vi "界面3.vi"() -> ()   [LabVIEW 2014]
uses:
  <vilib>/Analysis/3filter.llb/Filter Passband Type.ctl
  <vilib>/Analysis/4window.llb/windowTd.ctl
  <vilib>/Platform/TimedLoop/XDataNode/timing_clust.ctl
  <vilib>/Platform/TimedLoop/XDataNode/nitl_modes.ctl
  <vilib>/Platform/TimedLoop/XDataNode/wakeup.ctl
  <vilib>/Utility/error.llb/DialogType.ctl
  <vilib>/DAQmx/read.llb/DAQmx Read (Analog 1D Wfm NChan NSamp).vi
  <vilib>/express/express analysis/Spectral/Block/exnSpectralBlock spectral measurements peak poly.vi
  <vilib>/express/express analysis/Spectral/Block/exnSpectralBlock spectral measurements peak array WFM.vi
  <vilib>/express/express analysis/Spectral/Block/exnSpectralBlock spectral measurements peak WFM.vi
  <vilib>/DAQmx/create/channels.llb/DAQmx Create Channel (AI-Voltage-Basic).vi
  <vilib>/DAQmx/configure/timing.llb/DAQmx Timing (Sample Clock).vi
  <vilib>/DAQmx/miscellaneous.llb/DAQmx Fill In Error Info.vi
  <vilib>/Waveform/WDTOps.llb/WDT Number of Waveform Samples DBL.vi
  <vilib>/Waveform/WDTOps.llb/WDT Append Waveforms DBL.vi
  <vilib>/Waveform/WDTOps.llb/WDT Get Waveform Subset DBL.vi
  <vilib>/measure/macond.llb/IIR Filter for 1 Chan.vi
  <vilib>/express/express analysis/Spectral/XNode/ExpressSpectralMeasurementsBlockNode.xnode
  <vilib>/Platform/TimedLoop/XDataNode/XDataNode.xnode
  <vilib>/Platform/TimedLoop/XDataNode/XDNodeRunTimeDep.lvlib
  <vilib>/measure/NI_MAPro.lvlib
  <vilib>/Analysis/NI_AALBase.lvlib
  <vilib>/Analysis/NI_AALPro.lvlib
panel:
  out "主轴实际转速":dbl format="%#_g r/min"
  out "后端配重信号相位":dbl
  out "前端配重信号相位":dbl
  out "后端试重信号相位":dbl
  out "前端试重信号相位":dbl
  out "后端原始信号相位":dbl
  out "前端原始信号相位":dbl
  out "后端配重信号幅值":dbl
  out "前端配重信号幅值":dbl
  out "后端试重信号幅值":dbl
  out "前端试重信号幅值":dbl
  out "后端原始信号幅值":dbl
  out "前端原始信号幅值":dbl
  out "布尔":bool
  in  "?":enum32{"参数设置", " 数据采集", "振动分析", "试重平衡", "无试重平衡"}(tab)
  in  "传感器灵敏度 8":dbl=200.0 format="%#_g  μm/v"
  in  "传感器灵敏度 7":dbl=200.0 format="%#_g  μm/v"
  in  "传感器灵敏度 6":dbl=200.0 format="%#_g  μm/v"
  in  "传感器灵敏度 5":dbl=1.0 format="%#_g  μm/v"
  in  "传感器灵敏度 4":dbl=200.0 format="%#_g  μm/v"
  in  "传感器灵敏度 3":dbl=200.0 format="%#_g  μm/v"
  in  "传感器灵敏度 2":dbl=200.0 format="%#_g  μm/v"
  in  "滤波模式 2":T1(ring)
  in  "通道波形选择 2":T2(ring)
  in  "轴与传感器间的阈值距离":dbl=1000.0 caption="传感器与轴的阈值距离" format="%#_g  μm"
  in  "采样时间":dbl=200.0 format="%#_g  s"
  in  "主轴转速":dbl=200.0 format="%#_g  r/min"
  in  "传感器灵敏度":dbl=200.0 format="%#_g  μm/v"
  in  "rate":dbl=1000.0 caption="采样速率" format="%0.2f  HZ"
  in  "units":i32(ring)=10348 caption="采集电压单位" items=["伏特"=10348, "来自自定义换算"=10065]
  in  "number of samples per channel":i32=1000 caption="每通道采样数"
  in  "input terminal configuration":i32(ring)=-1 caption="输入接线端配置" items=["默认"=-1, "RSE"=10083, "NRSE"=10078, "差分"=10106, "伪差分"=12529]
  in  "最小采集电压值":dbl=-10.0 format="%#_g  V"
  in  "最大采集电压值":dbl=10.0 format="%#_g  V"
  in  "sample mode":i32(ring)=10178 caption="采样模式" items=["有限采样"=10178, "连续采样"=10123, "硬件定时单点"=12522]
  in  "通道":string(combo)="4"
  in  "转速阈值":dbl=10.0
  out "当前时间":timestamp format="%<%X\n%x>T"
  in  "电压&幅值":enum16{"电压", "幅值"}(ring)
  out "轴与传感器间的阈值距离":dbl format="%#_g  μm"
  out "采样时间":dbl format="%#_g  s"
  in  "?":bool
  in  "?":bool
  in  "?":bool
  out "主轴转速":dbl format="%#_g  r/min"
  out "传感器灵敏度":dbl format="%#_g  μm/V"
  in  "设置按钮":bool
  out "样本大小":dbl
  out "采样频率":dbl format="%#_g HZ"
  out "工频 8":dbl format="%0.2f  HZ"
  out "工频幅值 8":dbl format="%0.2f  μm"
  out "工频相位 8":dbl format="%0.2f  rad "
  out "工频 7":dbl format="%0.2f  HZ"
  out "工频幅值 7":dbl format="%0.2f  μm"
  out "工频相位 7":dbl format="%0.2f  rad "
  out "工频 6":dbl format="%0.2f  HZ"
  out "工频幅值 6":dbl format="%0.2f  μm"
  out "工频相位 6":dbl format="%0.2f  rad "
  out "工频 5":dbl format="%0.2f  HZ"
  out "工频幅值 5":dbl format="%0.2f  μm"
  out "工频相位 5":dbl format="%0.2f  rad "
  out "工频 4":dbl format="%0.2f  HZ"
  out "工频幅值 4":dbl format="%0.2f  μm"
  out "工频相位 4":dbl format="%0.2f  rad "
  out "工频 3":dbl format="%0.2f  HZ"
  out "工频幅值 3":dbl format="%0.2f  μm"
  out "工频相位 3":dbl format="%0.2f  rad"
  out "工频 2":dbl format="%0.2f  HZ"
  out "工频幅值 2":dbl format="%0.2f  μm"
  out "工频相位 2":dbl format="%0.2f  rad"
  in  "?":u32(colorbox)=16777222
  in  "?":u32(colorbox)=13132800
  in  "?":u32(colorbox)=12255487
  in  "?":u32(colorbox)=18175
  in  "?":u32(colorbox)=6618880
  in  "?":u32(colorbox)=16775281
  in  "?":u32(colorbox)=16717330
  out "时域波形图":waveform(dbl)[](graph)
  out "频域波形图":cluster{"f0":dbl, "df":dbl, "magnitude":dbl[]}[](graph)
  in  "physical channels 8":tag="Dev1/ai7" caption="物理通道8"
  in  "physical channels 7":tag="Dev1/ai6" caption="物理通道7"
  in  "physical channels 6":tag="Dev1/ai5" caption="物理通道6"
  in  "physical channels 5":tag="Dev1/ai4" caption="物理通道5"
  in  "physical channels 4":tag="Dev1/ai3" caption="物理通道4"
  in  "physical channels 3":tag="Dev1/ai2" caption="物理通道3"
  in  "physical channels 2":tag="Dev1/ai1" caption="物理通道2"
  in  "physical channels":tag="Dev1/ai0" caption="物理通道1"
  in  "?":bool
  in  "?":bool
  in  "?":bool
  in  "?":bool
  in  "?":bool
  in  "?":bool
  in  "?":bool
  in  "?":bool
  in  "?":u32(colorbox)=4385023
  out "传感器与轴的距离":u64
  out "传感器与轴的距离 8":u64
  out "传感器与轴的距离 2":u64
  out "传感器与轴的距离 3":u64
  out "传感器与轴的距离 4":u64
  out "传感器与轴的距离 5":u64
  out "传感器与轴的距离 6":u64
  out "传感器与轴的距离 7":u64
  out "工频（HZ）":dbl format="%0.2f  HZ"
  out "工频幅值（μm）":dbl format="%0.2f  μm"
  out "工频相位（rad）":dbl format="%0.2f rad"
  out "起始点":dbl
  in  "是否截取信号":bool
  in  "?":enum32{"数据滤波", "轴心轨迹", " 模态分析"}(tab)
  out "工频相位":dbl format="%0.2f  rad"
  out "工频幅值":dbl format="%0.2f  μm"
  out "工频频率":dbl format="%0.2f  HZ"
  in  "选项卡控件3":T3(tab)
  in  "高频截止频率":dbl(slide) scale=0.0..500.0
  in  "阶数":i32
  in  "低频截止频率":dbl(slide) scale=0.0..500.0
  in  "filter type":T4 caption="滤波器类型"
  in  "垂直指针滑动杆":dbl(slide) scale=0.0..100.0
  in  "参数设置按钮 2":bool
  out "滤波后频域信号":cluster{"f0":dbl, "df":dbl, "magnitude":dbl[]}(graph)
  out "滤波前频域信号":cluster{"f0":dbl, "df":dbl, "magnitude":dbl[]}(graph)
  out "滤波模式":T1(ring)
  out "滤波后时域信号":waveform(dbl)(graph)
  out "滤波前时域信号":waveform(dbl)(graph)
  out "通道波形选择":T2(ring)
  in  "电压&幅值 2":enum16{"电压", "幅值"}(ring)
  in  "保存轴心轨迹数据":bool
  out "前端实时轴心轨迹":cluster{"Array":dbl[], "Array":dbl[]}(graph)
  in  "?":string(combo)="1"
  in  "?":string(combo)="2"
  in  "3":string(combo)="3"
  in  "?":string(combo)="0"
  out "后端实时轴心轨迹":cluster{"Array":dbl[], "Array":dbl[]}(graph)
  in  "停止按钮":bool
  in  "预触发长度":i32
  in  "阈值设置":dbl=10.0 caption="阈值"
  in  "开始 3":bool
  in  "?":enum32{"时域信号", "频响函数信号"}(tab)
  out "激振信号":waveform(dbl)(graph)
  out "响应信号":waveform(dbl)(graph)={"t0"=timestamp(3578452120.913286 s since 1904-01-01), "dt"=0.001, "Y"=[]}
  in  "input terminal configuration 2":i32(ring)=-1 caption="输入接线端配置" items=["默认"=-1, "RSE"=10083, "NRSE"=10078, "差分"=10106, "伪差分"=12529]
  in  "rate 2":dbl=1000.0 caption="速率" format="%0.2f"
  in  "sample mode 2":i32(ring)=10178 caption="采样模式" items=["有限采样"=10178, "连续采样"=10123, "硬件定时单点"=12522]
  in  "number of samples per channel 2":i32=1000 caption="每通道采样数"
  in  "最小采集电压值 2":dbl=-10.0 format="%#_g  V"
  in  "最大采集电压值  2":dbl=10.0 format="%#_g  V"
  in  "采集次数":i32=3 caption="预触发长度"
  in  "units 3":i32(ring)=10348 caption="单位" items=["伏特"=10348, "来自自定义换算"=10065]
  out "相关函数":cluster{"f0":dbl, "df":dbl, "magnitude":dbl[]}(graph)
  out "FRF Phase":cluster{"f0":dbl, "df":dbl, "magnitude":dbl[]}(graph)
  out "FRF magnifitude":cluster{"f0":dbl, "df":dbl, "magnitude":dbl[]}(graph)
  out "模态振型":dbl[](array[numeric])
  out "固有频率":dbl[](array[numeric])
  out "模态阻尼比":dbl[](array[numeric])
  in  "激振通道":enum16{"激振信号", "响应信号"}(ring)
  in  "激振计数":i32 caption="预触发长度" format="%d /3"
  in  "averaging parameters":T5={"averaging mode"=enum."No averaging", "weighting mode"=enum."Exponential", "number of averages"=10} caption="平均参数" {"number of averages" min=1}
  in  "window":T6=1 caption="窗" items=["矩形"=0, "Hanning"=1, "Hamming"=2, "Blackman-Harris"=3, "Exact Blackman"=4, "Blackman"=5, "Flat Top"=6, "4阶Blackman-Harris "=7, "7阶Blackman-Harris"=8, "Low Sidelobe"=9, "Blackman Nuttall"=11, "三角"=30, "Bartlett-Hanning"=31, "Bohman"=32, "Parzen"=33, "Welch"=34, "Kaiser"=60, "Dolph-Chebyshev"=61, "高斯"=62]
  in  "view":T7 caption="查看"
  in  "FRF Mode":enum16{"H1", "H2", "H3"}(ring) caption="FRF模式"
  in  "删除上一次波形":bool
  in  "激振信号物理通道":tag="Dev1/ai0"
  in  "激振传感器灵敏度":dbl=1.0
  in  "响应信号物理通道":tag="Dev1/ai1"
  in  "响应传感器灵敏度":dbl=1.0 caption="激振传感器灵敏度"
  in  "模态阶数":i32
  in  "Lower Fc":dbl=1000.0
  in  "Order":i32=5
  out "时间间隔":dbl=0.01
  in  "后端":bool
  in  "前端":bool
  in  "配重盘孔数":dbl=16.0
  out "配重误差":dbl format="配重误差：%0.2f "
  in  "确定计算":bool
  out "第一配重重量":dbl format="第一配重重量：%0.2f g"
  out "第一配重位置":dbl format="第一配重位置：%0.1f 孔"
  out "第二配重重量":dbl format="第二配重重量：%0.2f g"
  out "第二配重位置":dbl format="第二配重位置：%0.1f 孔"
  out "配重信号相位":dbl format="Phase  %0.4f °"
  out "配重振动幅值":dbl format="Amp %0.4f μm"
  in  "配重信号":bool
  in  "试重信号":bool
  in  "试重位置":dbl format="试重位置：%0.1f 孔"
  in  "试重重量":dbl format="试重重量：%0.2f g"
  out "试重信号相位":dbl format="Phase %0.4f °"
  out "试重振动幅值":dbl format="Amp  %0.4f μm"
  out "原始信号相位":dbl format="Phase  %0.4f °"
  out "原始振动幅值":dbl format="Amp %0.4f μm"
  in  "刷新按钮 3":bool
  in  "刷新按钮 2":bool
  in  "刷新按钮":bool
  out "计数 2":i32
  out "计数3":i32
  out "计数":i32
  out "后端配重信号重组":cdb
  out "前端配重信号重组":cdb
  out "后端试重信号重组":cdb
  out "前端试重信号重组":cdb
  out "前端原始信号重组":cdb
  out "后端原始信号重组":cdb
  in  "冗余次数":i32
  out "频域信号":cluster{"f0":dbl, "df":dbl, "magnitude":dbl[]}[](graph)
  out "时域信号":waveform(dbl)[](graph)
  in  "开始 2":bool
  in  "?":string(combo)="0"
  in  "原始信号":bool
  in  "?":string(combo)="1"
  in  "?":string(combo)="2"
  in  "?":string(combo)="3"
  in  "?":bool
  in  "?":bool
  in  "?":bool
  in  "?":bool
  in  "?":string(combo)="1"
  in  "?":string(combo)="0"
  in  "高速主轴不平衡振动识别":bool
  in  "高速主轴不平衡振动行为分析":bool
  in  "高速主轴系统有限元动力学建模":bool
  in  "角接触球轴承有限元动力学建模":bool
  out "?":string
  # "转子动平衡测控系统"
  # "采集通道参数设置"
  # "外部硬件参数设置"
  # "传感器灵敏度参数设置"
  # "转速及相位信号参数设置"
  # "数据滤波参数设置"
  # "μm"
  # "通道一"
  # "μm"
  # "通道二"
  # "μm"
  # "通道三"
  # "μm"
  # "通道四"
  # "μm"
  # "通道五"
  # "μm"
  # "通道六"
  # "μm"
  # "通道七"
  # "μm"
  # "通道八"
  # "对应滤波模式参数设置"
  # "Butterworth\n Filter"
  # "前端信号通道选择"
  # "X轴"
  # "Y轴"
  # "后端信号通道选择"
  # "X轴"
  # "Y轴"
  # "低通时域滤波"
  # "求解频响函数参数设置"
  # "采集设置"
  # "选择进行动平衡的信号通道"
  # "前端X"
  # "前端Y"
  # "后端X"
  # "后端Y"
  # "选择实际\n试重平衡\n所需通道"
  # "计算配重"
  # "参考路径:E:\\matlab GUI\\gzkj"
  # "参考路径:E:\\matlab GUI\\gzkj"
  # "参考路径:E:\\matlab GUI\\zhendongfenxi"
  # "参考路径:E:\\matlab GUI\\bphxysb"
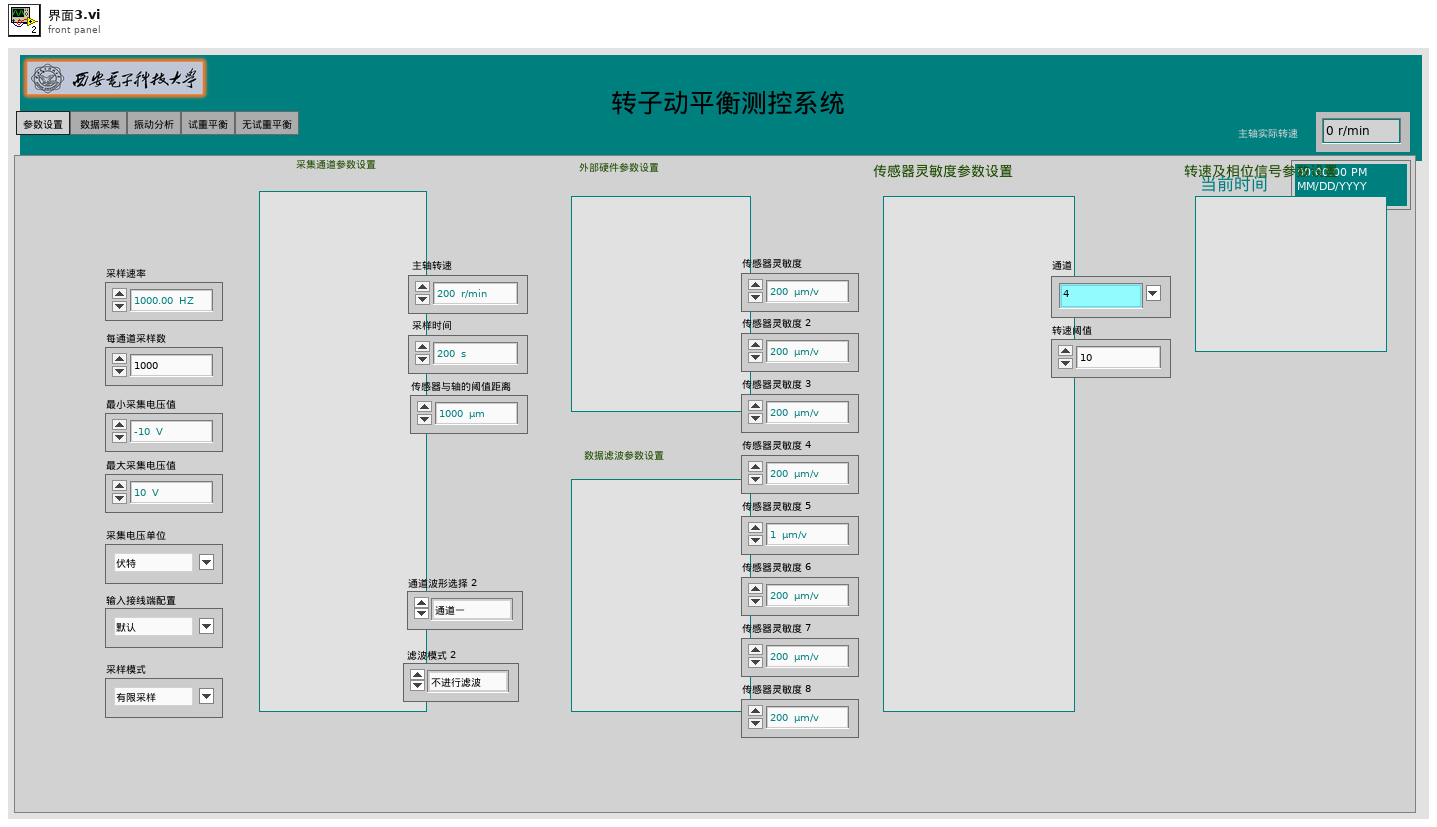
[diagram p1: front panel]
types:
  T1 = enum16{"不进行滤波", "FFT", "STFT", "自适应滤波", "小波包分解", "自己设计的滤波方法"}
  T2 = enum16{"通道一", "通道二", "通道三", "通道四", "通道五", "通道六", "通道七", "通道八"}
  T3 = enum32{"FFT", "STFT", "自适应滤波", "小波包分解", "by yourself "}
  T4 = typedef "NI_AALBase.lvlib/Filter Passband Type.ctl" = enum32{"Lowpass", "Highpass", "Bandpass", "Bandstop"}
  T5 = cluster{"averaging mode":enum16{"No averaging", "Vector averaging", "RMS averaging", "Peak hold"}, "weighting mode":enum16{"Linear", "Exponential"}, "number of averages":u32}
  T6 = typedef "NI_AALPro.lvlib/windowTd.ctl" = u32
  T7 = cluster{"dB On (F)":bool, "unwrap phase (F)":bool, "convert to degree (F)":bool}
  T8 = typedef "XDNodeRunTimeDep.lvlib/timing_clust.ctl" = cluster{"Expected End [f-1]":u64, "Actual End [f-1]":u64, "Finished Late? [f-1]":bool, "Expected End [i-1]":u64, "Actual End [i-1]":u64, "Finished Late? [i-1]":bool, "Expected Start [i]":u64, "Actual Start [i]":u64, "Expected Start [f]":u64, "Actual Start [f]":u64, "Source Name":string, "Structure Name":string, "Period":i64, "Deadline":i64, "Offset":i64, "Start":i64, "Priority":i32, "Timeout":i32, "Mode":T9, "Wakeup Reason":T10, "Error":errorcluster, "Source Type":string, "Secondary Source Type":string, "Global End Time":u64, "Global Start Time":u64, "Frame Duration":u64, "Iteration Duration":u64, "Assigned CPU":i32, "I/O Scan Engine Mode":u32}
  T9 = typedef "XDNodeRunTimeDep.lvlib/nitl_modes.ctl" = enum32{"No Change", "Process missed periods, maintain original phase", "Discard missed periods, maintain original phase", "Process missed periods, ignore original phase", "Discard missed periods, ignore original phase"}
  T10 = typedef "XDNodeRunTimeDep.lvlib/wakeup.ctl" = enum32{"Normal", "Aborted", "Asynchronous wakeup", "Timing source error", "Timed loop error", "Timeout"}
  T11 = cluster{"averaging mode":u16, "weighting mode":u16, "number of averages":u32}
  T12 = enum16{"Lowpass", "Highpass", "Bandpass", "Bandstop"}
  T13 = cluster{"Topology":enum16{"Off", "Butterworth", "Chebyshev", "Inverse Chebyshev", "Elliptic", "Bessel"}, "Type":enum16{"Lowpass", "Highpass", "Bandpass", "Bandstop"}, "Order":i32, "Lower Fc":dbl, "Upper Fc":dbl, "PB Ripple":dbl, "SB Attenuation":dbl}
  T14 = typedef "DialogType.ctl" = u16
  T15 = cluster{"magnitude":cluster{"f0":dbl, "df":dbl, "magnitude":dbl[]}, "phase":cluster{"f0":dbl, "df":dbl, "phase":dbl[]}, "coherence":cluster{"f0":dbl, "df":dbl, "coherence":dbl[]}}
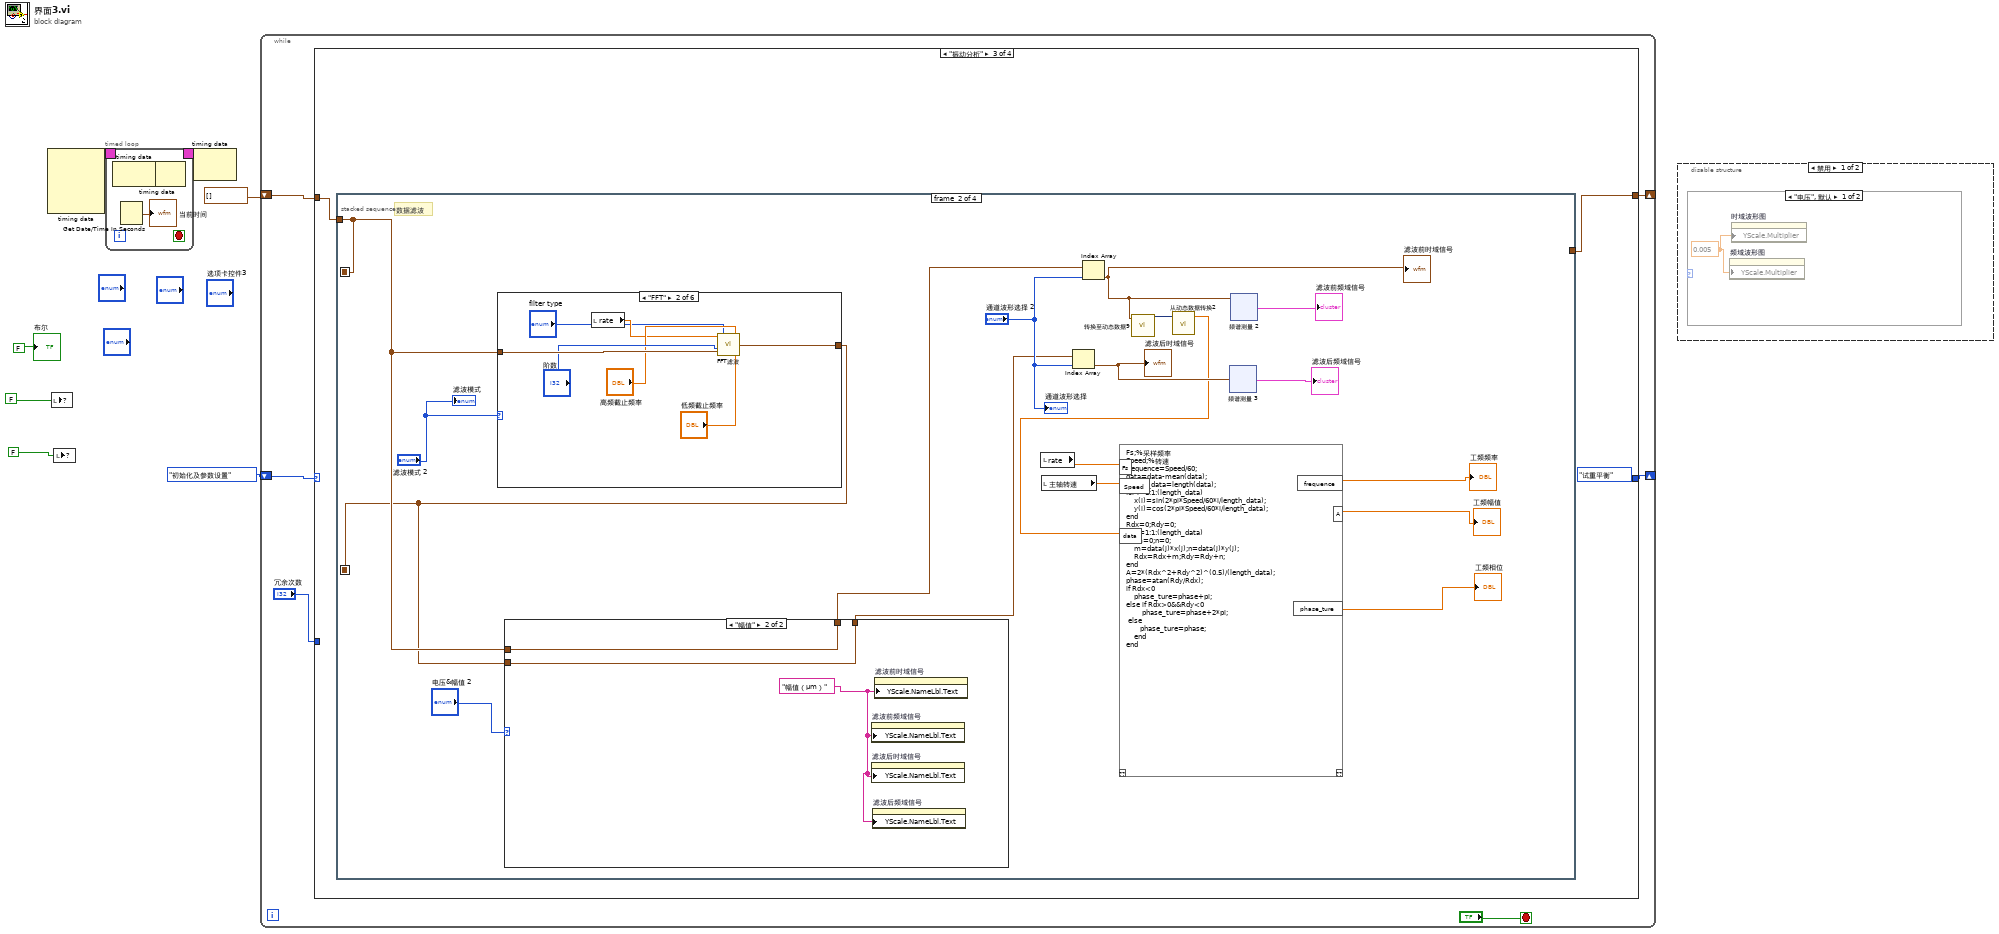
[diagram p0: block diagram]
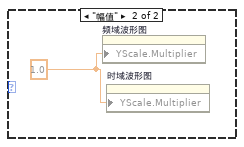
[diagram p2: hidden frame]
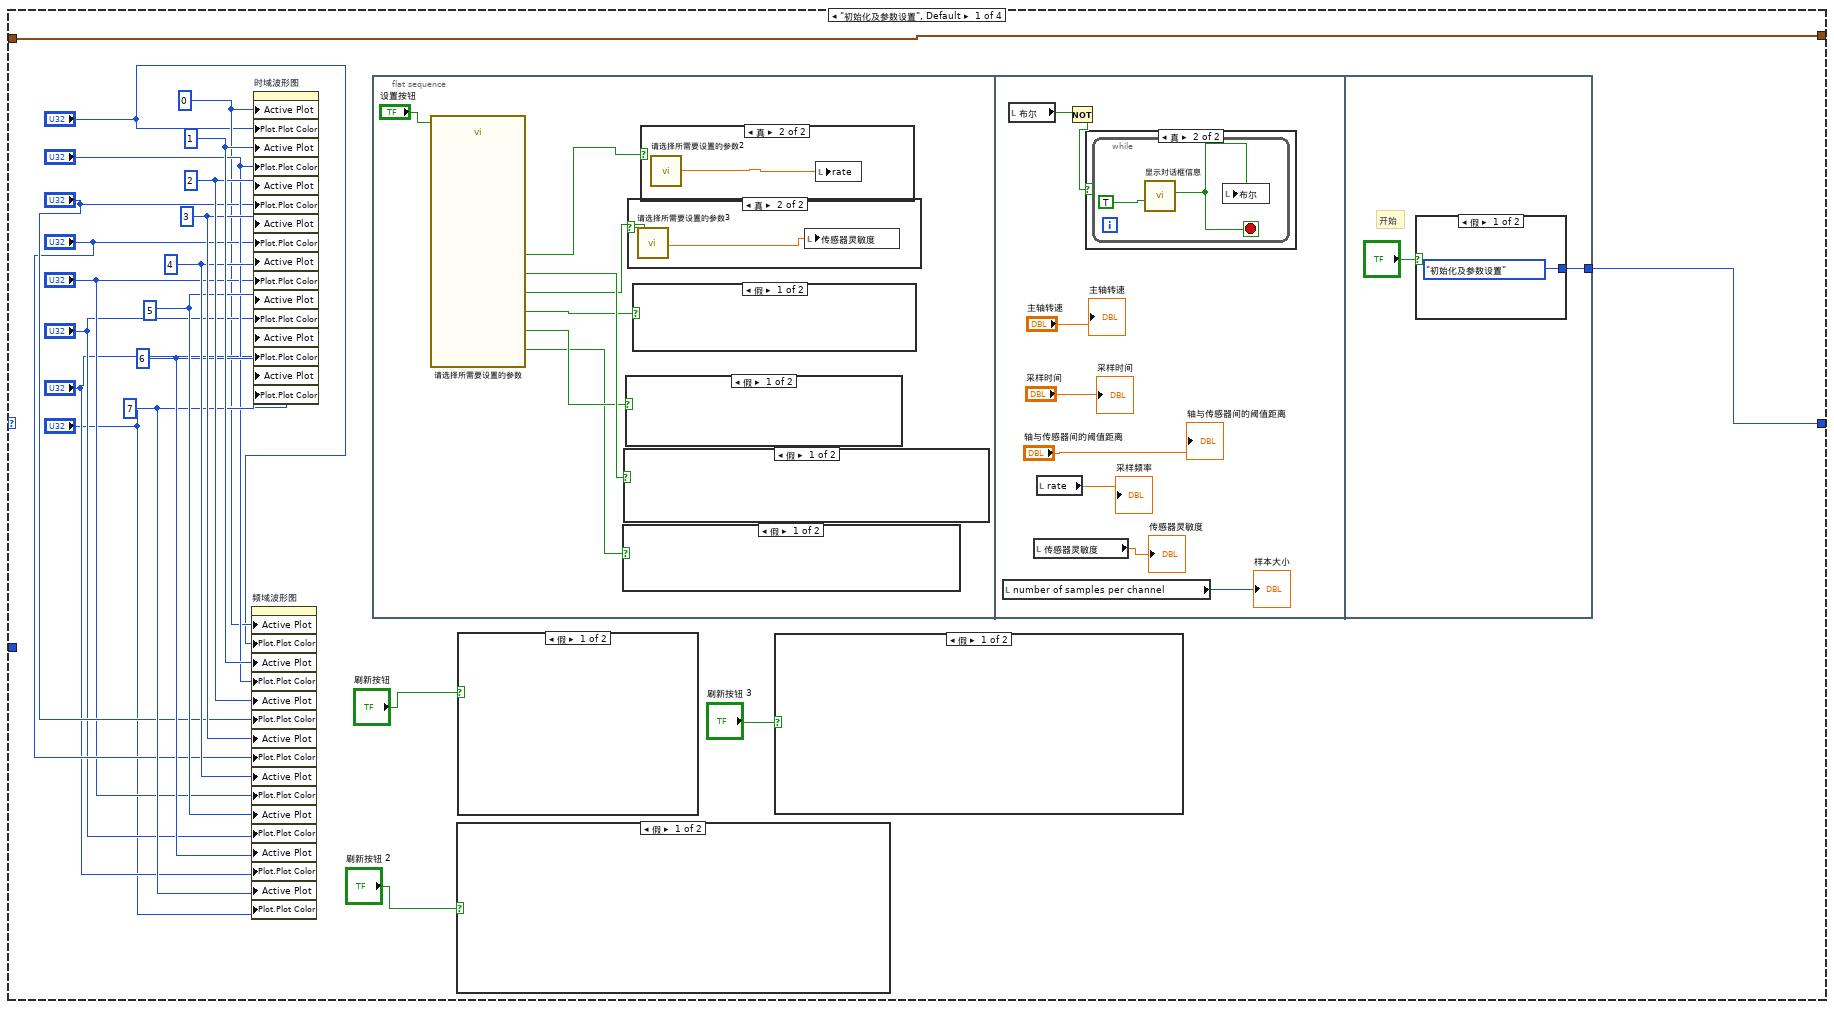
[diagram p4: hidden frame]
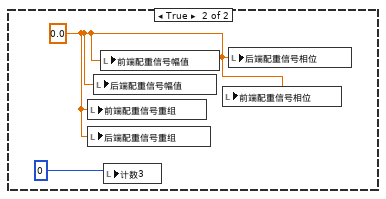
[diagram p5: hidden frame]
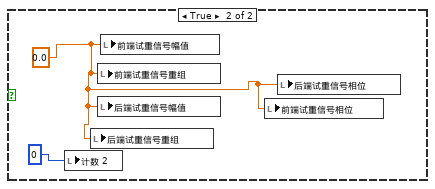
[diagram p6: hidden frame]
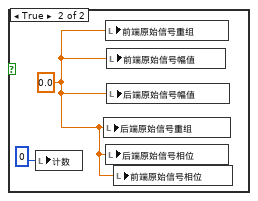
[diagram p7: hidden frame]
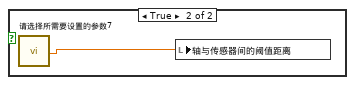
[diagram p8: hidden frame]
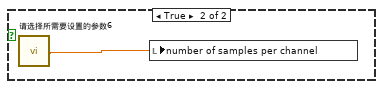
[diagram p9: hidden frame]
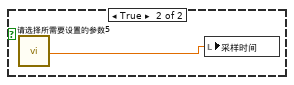
[diagram p10: hidden frame]
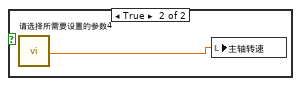
[diagram p11: hidden frame]
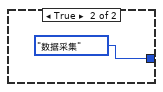
[diagram p15: hidden frame]
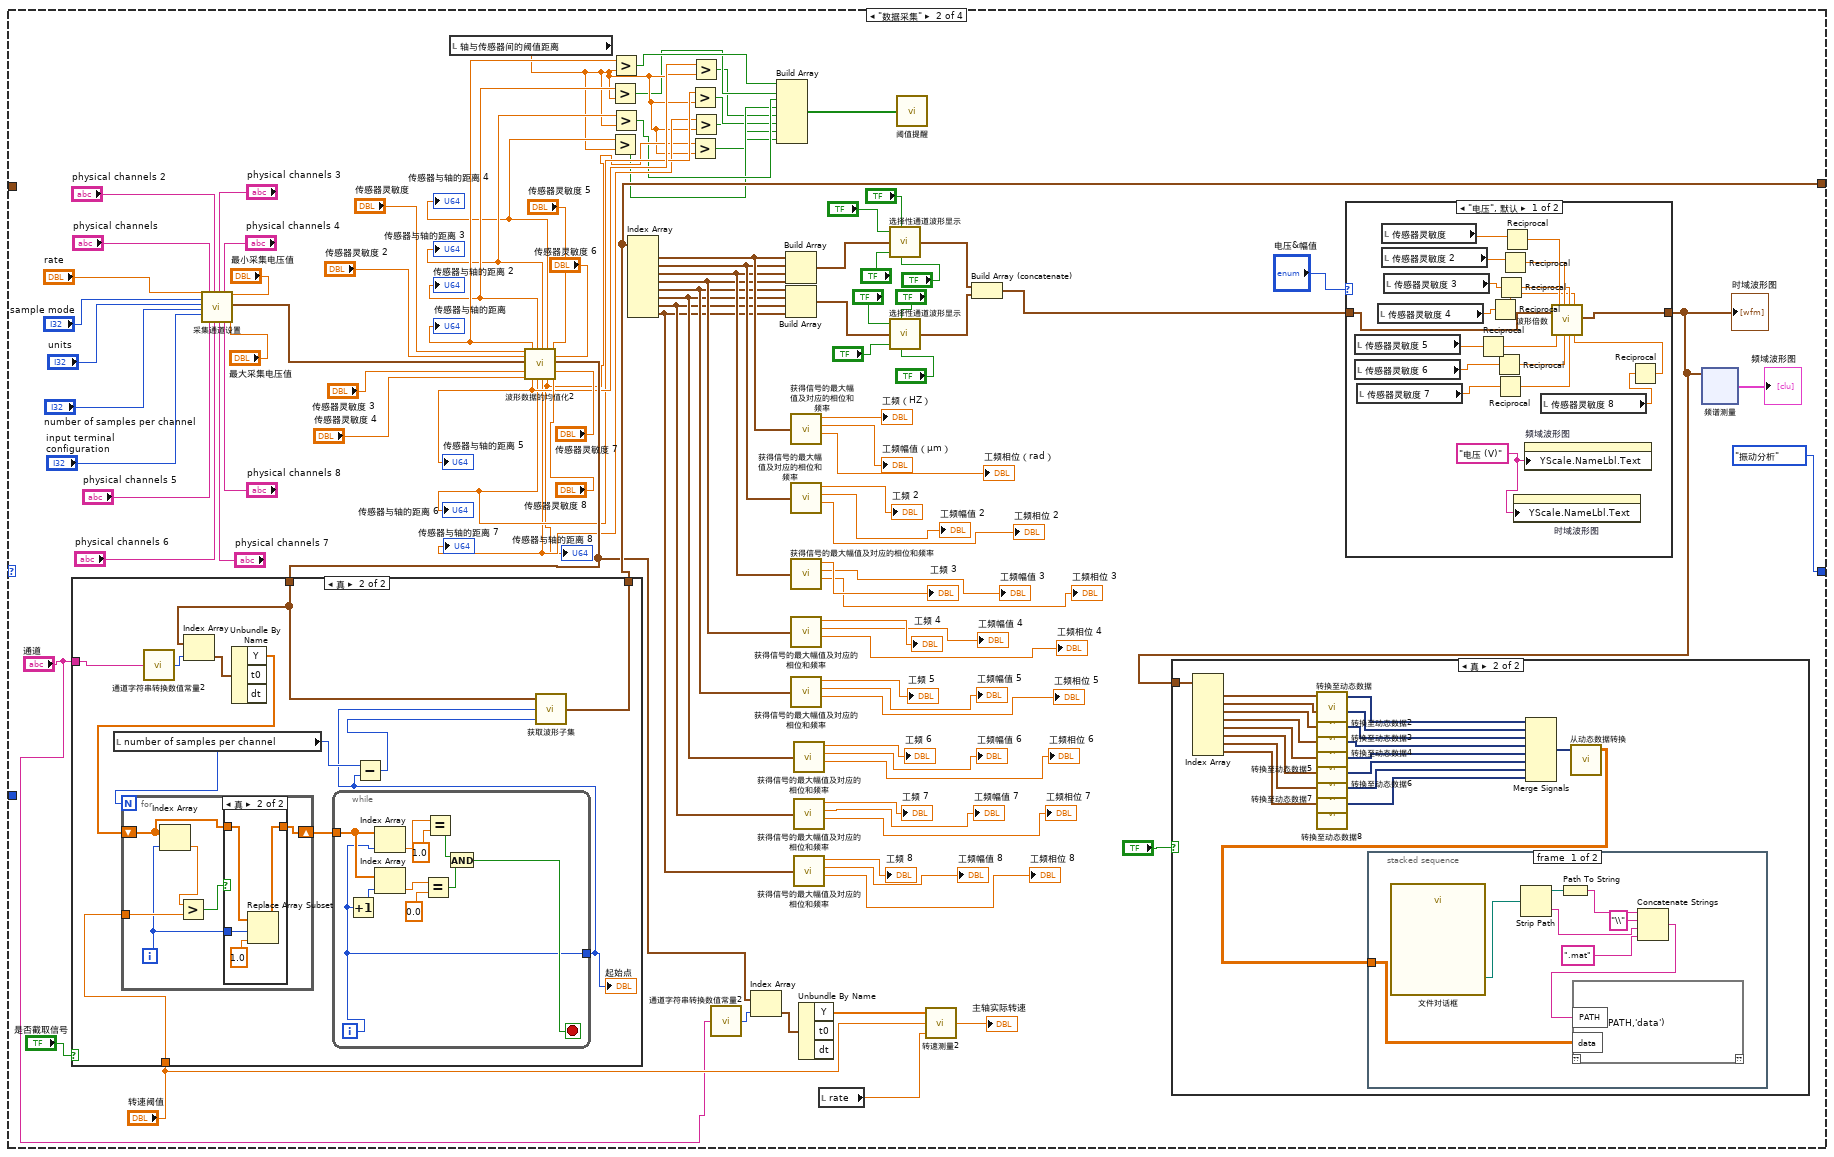
[diagram p16: hidden frame]
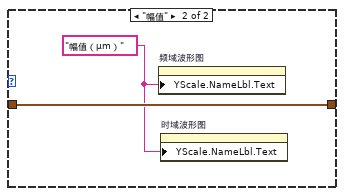
[diagram p17: hidden frame]
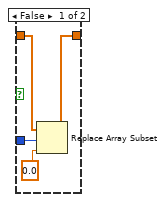
[diagram p19: hidden frame]
diagram:
  n1 = node-c288() -> (w7:T8)  [unwired: 4 in]
  n2 = local write item#75(FALSE) -> ()
  n3 = local write item#4(FALSE) -> ()
  n4 = timed-loop {
    timing: w7 -> [_]
    timing-out: [_] -> w6
    stop <- _ stop-if-true
    n5 = node-c288() -> ()  [unwired: 1 in, 1 out]
    n6 = Get Date/Time In Seconds() -> (seconds since 1Jan1904=→"当前时间":timestamp)
    n7 = node-c288() -> ()  [unwired: 1 in, 1 out]
  }
  n8 = node-c288(w6) -> ()  [unwired: 1 out]
  n9 = while {
    shift-right: [w12] -> _
    shift-left: enum16{"初始化及参数设置", "数据采集", "振动分析", "试重平衡"}."初始化及参数设置" -> [w15]
    shift-right: [w13] -> _
    shift-left: waveform(dbl)[] [] -> [w14]
    stop <- "?" stop-if-true
    n10 = case shown="\"振动分析\"" w15 {
      tunnel: w14 -> [w37 _ w271 w562]
      tunnel: [w37 w101 w270 w562] -> w13
      tunnel: [w20 enum16{"初始化及参数设置", "数据采集", "振动分析", "试重平衡"}."振动分析" ("枚举") enum16{"初始化及参数设置", "数据采集", "振动分析", "试重平衡"}."试重平衡" enum16{"初始化及参数设置", "数据采集", "振动分析", "试重平衡"}."初始化及参数设置"] -> w12
      tunnel: "冗余次数" -> [_ _ _ w564]
      frame "初始化及参数设置", Default {
        w30 = 7
        w31 = 6
        w32 = 5
        w33 = 4
        w34 = 3
        w35 = 2
        w36 = 1
        w22 = 0
        n11 = property on="频域波形图" class="WFGraph (严格)"("Active Plot"=w22, "Plot.Plot Color"="?", "Active Plot"=w36, "Plot.Plot Color"="?", "Active Plot"=w35, "Plot.Plot Color"="?", "Active Plot"=w34, "Plot.Plot Color"="?", "Active Plot"=w33, "Plot.Plot Color"="?", "Active Plot"=w32, "Plot.Plot Color"="?", "Active Plot"=w31, "Plot.Plot Color"="?", "Active Plot"=w30, "Plot.Plot Color"="?") -> ()  [unwired: 2 in, 2 out]
        n12 = property on="时域波形图" class="WFGraph (严格)"("Active Plot"=w22, "Plot.Plot Color"="?", "Active Plot"=w36, "Plot.Plot Color"="?", "Active Plot"=w35, "Plot.Plot Color"="?", "Active Plot"=w34, "Plot.Plot Color"="?", "Active Plot"=w33, "Plot.Plot Color"="?", "Active Plot"=w32, "Plot.Plot Color"="?", "Active Plot"=w31, "Plot.Plot Color"="?", "Active Plot"=w30, "Plot.Plot Color"="?") -> ()  [unwired: 2 in, 2 out]
        n13 = flat-sequence {
          tunnel: [w67] -> w20
          frame #0 {
            n14 = call "请选择所需要设置的参数"("Enable"="设置按钮") -> ("轴与传感器间的阈值距离（μm）"=w45:bool, "采样时间（s）"=w46:bool, "主轴转速（r/min）"=w47:bool, "传感器灵敏度（μm/v）"=w48:bool, "样本大小"=w49:bool, "采样频率"=w50:bool)  [unwired: 11 in, 2 out]
            n15 = case shown="假" w45 {
              frame False {
              }
              frame True {
                n16 = call "请选择所需要设置的参数7"() -> ("轴与传感器间的阈值距离（μm）"=w51:dbl)  [unwired: 17 in, 2 out]
                n17 = local write "轴与传感器间的阈值距离"(w51) -> ()
              }
            }
            n18 = case shown="假" w49 {
              frame False {
              }
              frame True {
                n19 = call "请选择所需要设置的参数6"() -> ("样本大小"=w52:dbl)  [unwired: 17 in, 2 out]
                n20 = local write "number of samples per channel"(w52) -> ()
              }
            }
            n21 = case shown="假" w46 {
              frame False {
              }
              frame True {
                n22 = call "请选择所需要设置的参数5"() -> ("采样时间（s）"=w53:dbl)  [unwired: 17 in, 2 out]
                n23 = local write "采样时间"(w53) -> ()
              }
            }
            n24 = case shown="真" w48 {
              frame False {
              }
              frame True {
                n25 = call "请选择所需要设置的参数3"() -> ("传感器灵敏度（μm/v）"=w55:dbl)  [unwired: 17 in, 2 out]
                n26 = local write "传感器灵敏度"(w55) -> ()
              }
            }
            n27 = case shown="假" w47 {
              frame False {
              }
              frame True {
                n28 = call "请选择所需要设置的参数4"() -> ("主轴转速（r/min）"=w54:dbl)  [unwired: 17 in, 2 out]
                n29 = local write "主轴转速"(w54) -> ()
              }
            }
            n30 = case shown="真" w50 {
              frame False {
              }
              frame True {
                n31 = call "请选择所需要设置的参数2"() -> ("采样频率"=w56:dbl)  [unwired: 17 in, 2 out]
                n32 = local write "rate"(w56) -> ()
              }
            }
          }
          frame #1 {
            n33 = local read "number of samples per channel"() -> (→"样本大小":i32)
            n34 = local read "布尔"() -> (w64:bool)
            n35 = local read "传感器灵敏度"() -> (→"传感器灵敏度":dbl)
            n36 = local read "rate"() -> (→"采样频率":dbl)
            n37 = Not(x=w64) -> (.not. x?=w63:bool)
            n38 = case shown="真" w63 {
              frame False {
              }
              frame True {
                n39 = while {
                  stop <- w65 stop-if-true
                  n40 = call "显示对话框信息"("Enable"=TRUE) -> ("确定"=w65:bool)  [unwired: 9 in, 1 out]
                  n41 = local write "布尔"(w65) -> ()
                }
              }
            }
            "主轴转速" <- "主轴转速"
            "采样时间" <- "采样时间"
            "轴与传感器间的阈值距离" <- "轴与传感器间的阈值距离"
          }
          frame #2 {
            # "开始"
            n42 = case shown="假" "?" {
              tunnel: [enum16{"初始化及参数设置", "数据采集", "振动分析", "试重平衡"}."初始化及参数设置" enum16{"初始化及参数设置", "数据采集", "振动分析", "试重平衡"}."数据采集"] -> w67
              frame False {
              }
              frame True {
              }
            }
          }
        }
        n43 = case shown="假" "刷新按钮 2" {
          frame False {
          }
          frame True {
            w40 = 0.0
            n44 = local write "计数 2"(0) -> ()
            n45 = local write "后端试重信号重组"(w40) -> ()
            n46 = local write "前端试重信号重组"(w40) -> ()
            n47 = local write "后端试重信号幅值"(w40) -> ()
            n48 = local write "前端试重信号幅值"(w40) -> ()
            n49 = local write "前端试重信号相位"(w40) -> ()
            n50 = local write "后端试重信号相位"(w40) -> ()
          }
        }
        n51 = case shown="假" "刷新按钮" {
          frame False {
          }
          frame True {
            w42 = 0.0
            n52 = local write "计数"(0) -> ()
            n53 = local write "后端原始信号重组"(w42) -> ()
            n54 = local write "前端原始信号重组"(w42) -> ()
            n55 = local write "后端原始信号相位"(w42) -> ()
            n56 = local write "前端原始信号幅值"(w42) -> ()
            n57 = local write "后端原始信号幅值"(w42) -> ()
            n58 = local write "前端原始信号相位"(w42) -> ()
          }
        }
        n59 = case shown="假" "刷新按钮 3" {
          frame False {
          }
          frame True {
            w38 = 0.0
            n60 = local write "前端配重信号重组"(w38) -> ()
            n61 = local write "后端配重信号重组"(w38) -> ()
            n62 = local write "后端配重信号幅值"(w38) -> ()
            n63 = local write "前端配重信号幅值"(w38) -> ()
            n64 = local write "计数3"(0) -> ()
            n65 = local write "前端配重信号相位"(w38) -> ()
            n66 = local write "后端配重信号相位"(w38) -> ()
          }
        }
      }
      frame "数据采集" {
        n67 = call "采集通道设置.vi"("rate"="rate", "sample mode"="sample mode", "units"="units", "number of samples per channel"="number of samples per channel", "input terminal configuration"="input terminal configuration", "physical channels"="physical channels", "physical channels 5"="physical channels 5", "physical channels 2"="physical channels 2", "physical channels 6"="physical channels 6", "physical channels 3"="physical channels 3", "physical channels 7"="physical channels 7", "physical channels 4"="physical channels 4", "physical channels 8"="physical channels 8", "最小采集电压值"="最小采集电压值", "最大采集电压值"="最大采集电压值") -> ("波形图"=w99:waveform(dbl)[])  [unwired: 4 in]
        n68 = local read "轴与传感器间的阈值距离"() -> (w80:dbl)
        n69 = call "波形数据的均值化2.vi"("传感器灵敏度"="传感器灵敏度", "传感器灵敏度 2"="传感器灵敏度 2", "温度信号"=w99, "传感器灵敏度 3"="传感器灵敏度 3", "传感器灵敏度 4"="传感器灵敏度 4", "传感器灵敏度 5"="传感器灵敏度 5", "传感器灵敏度 6"="传感器灵敏度 6", "传感器灵敏度 7"="传感器灵敏度 7", "传感器灵敏度 8"="传感器灵敏度 8") -> ("传感器与轴的距离"=w88:dbl, "传感器与轴的距离 5"=w84:dbl, "传感器与轴的距离 2"=w87:dbl, "传感器与轴的距离 6"=w83:dbl, "传感器与轴的距离 3"=w86:dbl, "传感器与轴的距离 7"=w82:dbl, "传感器与轴的距离 4"=w85:dbl, "传感器与轴的距离 8"=w81:dbl, "温度信号 3"=w90:waveform(dbl)[])  [unwired: 2 in]
        "传感器与轴的距离 2" <- w87
        "传感器与轴的距离 3" <- w86
        "传感器与轴的距离 4" <- w85
        "传感器与轴的距离 5" <- w84
        "传感器与轴的距离 6" <- w83
        "传感器与轴的距离 7" <- w82
        "传感器与轴的距离" <- w88
        "传感器与轴的距离 8" <- w81
        n70 = case shown="真" "是否截取信号" {
          tunnel: w90 -> [w194 w200]
          tunnel: [w194 w199] -> w101
          tunnel: "转速阈值" -> [_ w196]
          tunnel: "通道" -> [_ w195]
          frame False {
          }
          frame True {
            n71 = local read "number of samples per channel"() -> (w202:i32)
            n72 = call "通道字符串转换数值常量2.vi"(1:w195) -> ("数值"=w205:i32)
            n73 = Index Array(array=w200, index=w205) -> (element=w204:waveform(dbl))
            n74 = Unbundle By Name(w204) -> ("Y"=w198:dbl[])  [unwired: 2 out]
            n75 = for {
              N: w202 -> [_]
              shift-right: [w216] -> w203
              shift-left: w198 -> [w218]
              tunnel: w196 -> [w221]
              i -> [w217]
              n76 = Index Array(array=w218, index=w217) -> (element=w220:dbl)
              n77 = Greater?(x=w220, y=w221) -> (0:w219:bool)
              n78 = case shown="真" w219 {
                tunnel: w218 -> [w223 w229]
                tunnel: w217 -> [w225 w228]
                tunnel: [w222 w226] -> w216
                frame False {
                  n79 = Replace Array Subset(array=w223, new element=0.0, index=w225) -> (w222:dbl[])
                }
                frame True {
                  n80 = Replace Array Subset(array=w229, new element=1.0, index=w228) -> (w226:dbl[])
                }
              }
            }
            n81 = while {
              tunnel: w203 -> [w215]
              tunnel: [w206] -> w197
              i -> [w206]
              stop <- w207 stop-if-true
              n82 = Increment(x=w206) -> (x+1=w214:i32)
              n83 = Index Array(array=w215, index=w206) -> (element=w213:dbl)
              n84 = Index Array(array=w215, index=w214) -> (element=w210:dbl)
              n85 = Equal?(x=w210, y=0.0) -> (x = y?=w208:bool)
              n86 = Equal?(x=w213, y=1.0) -> (x = y?=w209:bool)
              n87 = And(x=w209, y=w208) -> (x .and. y?=w207:bool)
            }
            "起始点" <- w197
            n88 = Subtract(x=w202, y=w197) -> (x-y=w201:i32)
            n89 = call "获取波形子集.vi"("duration"=w201, "start samples/time"=w197, "时域波形图"=w200) -> ("时域波形图 2"=w199:waveform(dbl)[])
          }
        }
        n90 = Greater?(x=w87, y=w80) -> (0:w78:bool)
        n91 = Greater?(x=w85, y=w80) -> (0:w76:bool)
        n92 = Greater?(x=w88, y=w80) -> (0:w79:bool)
        n93 = Greater?(x=w86, y=w80) -> (0:w77:bool)
        n94 = Index Array(array=w101) -> (element #1=w144:waveform(dbl), element #2=w140:waveform(dbl), element #3=w136:waveform(dbl), element #4=w135:waveform(dbl), element #5=w134:waveform(dbl), element #6=w133:waveform(dbl), element #7=w132:waveform(dbl), element #8=w131:waveform(dbl))  [unwired: 8 in]
        n95 = Greater?(x=w83, y=w80) -> (0:w74:bool)
        n96 = Greater?(x=w81, y=w80) -> (0:w72:bool)
        n97 = Greater?(x=w84, y=w80) -> (0:w75:bool)
        n98 = Greater?(x=w82, y=w80) -> (0:w73:bool)
        n99 = call "通道字符串转换数值常量2.vi"(1:"通道") -> ("数值"=w97:i32)
        n100 = Index Array(array=w90, index=w97) -> (element=w96:waveform(dbl))
        n101 = Build Array(w79, w78, w77, w76, w75, w74, w73, w72) -> (w71:bool[])
        n102 = Build Array(w144, w140, w136, w135) -> (w156:waveform(dbl)[])
        n103 = Build Array(w134, w133, w132, w131) -> (w155:waveform(dbl)[])
        n104 = call "获得信号的最大幅值及对应的相位和频率.vi"("信号"=w144) -> ("max（f)"=→"工频（HZ）":dbl, "max幅值"=→"工频幅值（μm）":dbl, "max相位"=→"工频相位（rad）":dbl)  [unwired: 1 out]
        n105 = call "获得信号的最大幅值及对应的相位和频率.vi"("信号"=w140) -> ("max（f)"=→"工频 2":dbl, "max幅值"=→"工频幅值 2":dbl, "max相位"=→"工频相位 2":dbl)  [unwired: 1 out]
        n106 = call "获得信号的最大幅值及对应的相位和频率.vi"("信号"=w136) -> ("max（f)"=→"工频 3":dbl, "max幅值"=→"工频幅值 3":dbl, "max相位"=→"工频相位 3":dbl)  [unwired: 1 out]
        n107 = call "获得信号的最大幅值及对应的相位和频率.vi"("信号"=w135) -> ("max（f)"=→"工频 4":dbl, "max幅值"=→"工频幅值 4":dbl, "max相位"=→"工频相位 4":dbl)  [unwired: 1 out]
        n108 = call "获得信号的最大幅值及对应的相位和频率.vi"("信号"=w134) -> ("max（f)"=→"工频 5":dbl, "max幅值"=→"工频幅值 5":dbl, "max相位"=→"工频相位 5":dbl)  [unwired: 1 out]
        n109 = call "获得信号的最大幅值及对应的相位和频率.vi"("信号"=w133) -> ("max（f)"=→"工频 6":dbl, "max幅值"=→"工频幅值 6":dbl, "max相位"=→"工频相位 6":dbl)  [unwired: 1 out]
        n110 = call "获得信号的最大幅值及对应的相位和频率.vi"("信号"=w132) -> ("max（f)"=→"工频 7":dbl, "max幅值"=→"工频幅值 7":dbl, "max相位"=→"工频相位 7":dbl)  [unwired: 1 out]
        n111 = call "获得信号的最大幅值及对应的相位和频率.vi"("信号"=w131) -> ("max（f)"=→"工频 8":dbl, "max幅值"=→"工频幅值 8":dbl, "max相位"=→"工频相位 8":dbl)  [unwired: 1 out]
        n112 = Unbundle By Name(w96) -> ("Y"=w94:dbl[])  [unwired: 2 out]
        n113 = local read "rate"() -> (w93:dbl)
        n114 = call "选择性通道波形显示.vi"("布尔"="?", "布尔 2"="?", "振动信号"=w156, "布尔 3"="?", "布尔 4"="?") -> ("选择性显示通道信号"=w146:waveform(dbl)[])  [unwired: 4 in]
        n115 = call "选择性通道波形显示.vi"("布尔"="?", "布尔 2"="?", "振动信号"=w155, "布尔 3"="?", "布尔 4"="?") -> ("选择性显示通道信号"=w145:waveform(dbl)[])  [unwired: 4 in]
        n116 = call "阈值提醒.vi"("添加的数组"=w71) -> ()
        n117 = call "转速测量2.vi"("采样频率"=w93, "阈值"="转速阈值", "转速数组"=w94) -> ("转速"=→"主轴实际转速":dbl)
        n118 = Build Array (concatenate)(w146, w145) -> (w98:waveform(dbl)[])
        n119 = case shown="\"电压\", 默认" "电压&幅值" {
          tunnel: w98 -> [w191 w193]
          tunnel: [w190 w193] -> w89
          frame "电压", Default {
            w173 = "电压 (V)"
            n120 = local read "传感器灵敏度 5"() -> (w181:dbl)
            n121 = local read "传感器灵敏度 6"() -> (w179:dbl)
            n122 = local read "传感器灵敏度 7"() -> (w178:dbl)
            n123 = local read "传感器灵敏度 4"() -> (w183:dbl)
            n124 = local read "传感器灵敏度"() -> (w189:dbl)
            n125 = local read "传感器灵敏度 2"() -> (w187:dbl)
            n126 = local read "传感器灵敏度 3"() -> (w185:dbl)
            n127 = Reciprocal(x=w181) -> (1/x=w180:dbl)
            n128 = Reciprocal(x=w183) -> (1/x=w182:dbl)
            n129 = Reciprocal(x=w179) -> (1/x=w177:dbl)
            n130 = Reciprocal(x=w178) -> (1/x=w176:dbl)
            n131 = Reciprocal(x=w185) -> (1/x=w184:dbl)
            n132 = Reciprocal(x=w187) -> (1/x=w186:dbl)
            n133 = Reciprocal(x=w189) -> (1/x=w188:dbl)
            n134 = property on="时域波形图" class="WFGraph (严格)"("YScale.NameLbl.Text"=w173) -> ()  [unwired: 2 in, 2 out]
            n135 = property on="频域波形图" class="WFGraph (严格)"("YScale.NameLbl.Text"=w173) -> ()  [unwired: 2 in, 2 out]
            n136 = local read "传感器灵敏度 8"() -> (w175:dbl)
            n137 = Reciprocal(x=w175) -> (1/x=w174:dbl)
            n138 = call "波形倍数.vi"("时域波形图"=w191, "数值"=w188, "数值 5"=w180, "数值 2"=w186, "数值 6"=w177, "数值 3"=w184, "数值 7"=w176, "数值 4"=w182, "数值 8"=w174) -> ("时域波形图 2"=w190:waveform(dbl)[])  [unwired: 10 in]
          }
          frame "幅值" {
            w192 = "幅值（μm）"
            n139 = property on="频域波形图" class="WFGraph (严格)"("YScale.NameLbl.Text"=w192) -> ()  [unwired: 2 in, 2 out]
            n140 = property on="时域波形图" class="WFGraph (严格)"("YScale.NameLbl.Text"=w192) -> ()  [unwired: 2 in, 2 out]
          }
        }
        "时域波形图" <- w89
        n141 = case shown="真" "?" {
          tunnel: w89 -> [_ w248]
          frame False {
          }
          frame True {
            n142 = Index Array(array=w248) -> (element #1=w247:waveform(dbl), element #2=w246:waveform(dbl), element #3=w245:waveform(dbl), element #4=w244:waveform(dbl), element #5=w243:waveform(dbl), element #6=w242:waveform(dbl), element #7=w241:waveform(dbl), element #8=w240:waveform(dbl))  [unwired: 8 in]
            n143 = call "转换至动态数据"("Waveform"=w247) -> ("Dynamic Data Type"=w239:dynamicdata)  [unwired: 3 in]
            n144 = call "转换至动态数据2"("Waveform"=w246) -> ("Dynamic Data Type"=w238:dynamicdata)  [unwired: 3 in]
            n145 = call "转换至动态数据3"("Waveform"=w245) -> ("Dynamic Data Type"=w237:dynamicdata)  [unwired: 3 in]
            n146 = call "转换至动态数据4"("Waveform"=w244) -> ("Dynamic Data Type"=w236:dynamicdata)  [unwired: 3 in]
            n147 = call "转换至动态数据5"("Waveform"=w243) -> ("Dynamic Data Type"=w235:dynamicdata)  [unwired: 3 in]
            n148 = call "转换至动态数据6"("Waveform"=w242) -> ("Dynamic Data Type"=w234:dynamicdata)  [unwired: 3 in]
            n149 = call "转换至动态数据7"("Waveform"=w241) -> ("Dynamic Data Type"=w233:dynamicdata)  [unwired: 3 in]
            n150 = call "转换至动态数据8"("Waveform"=w240) -> ("Dynamic Data Type"=w232:dynamicdata)  [unwired: 3 in]
            n151 = Merge Signals(w239, w238, w237, w236, w235, w234, w233, w232) -> (w231:dynamicdata)
            n152 = call "从动态数据转换"("Dynamic Data Type"=w231) -> ("Array"=w230:dbl[][])  [unwired: 3 in]
            n153 = stacked-sequence {
              tunnel: w230 -> [w250 _]
              frame #0 {
                n154 = call "文件对话框"() -> ("selected path"=w256:path)  [unwired: 12 in, 3 out]
                n155 = Strip Path(path=w256) -> (stripped path=w252:path, name=w251:string)
                n156 = Path To String(path=w252) -> (string=w255:string)
                n157 = Concatenate Strings(w255, "\\" ("字符串"), w251, ".mat" ("字符串")) -> (w249:string)
                n158 = script code="save(PATH,'data')"("PATH"=w249, "data"=w250) -> ()  [unwired: 1 in, 1 out]
              }
              frame #1 {
                n159 = call "显示对话框信息2"("Enable"=TRUE) -> ("确定"=w258:bool)  [unwired: 9 in, 1 out]
                n160 = Not(x=w258) -> (.not. x?=w257:bool)
                n161 = local write item#75(w257) -> ()
              }
            }
          }
        }
        n162 = xnode "频谱测量"("信号"=w89) -> ("FFT - （峰值）"=→"频域波形图":cluster{"f0":dbl, "df":dbl, "magnitude":dbl[]}[])  [unwired: 1 in, 2 out]
      }
      frame "振动分析" {
        n163 = stacked-sequence {
          seq-local: [_ w301 _ _] -> [_ _ w382 _]
          seq-local: [_ w302 _ _] -> [_ _ w377 _]
          tunnel: w271 -> [_ w302 _ _]
          tunnel: [_ _ w377 _] -> w270
          frame #0 {
            # "参数设置"
            n164 = case shown="真" "参数设置按钮 2" {
              selector: "参数设置按钮 2" -> [_ w276]
              frame False {
              }
              frame True {
                n165 = call "请选择数据处理参数设置"("Enable"=w276) -> ("滤波模式选择"=w275:bool, "通道选择"=w274:bool)  [unwired: 15 in, 2 out]
                n166 = case shown="真" w274 {
                  selector: w274 -> [_ w288]
                  frame False {
                  }
                  frame True {
                    n167 = call "请选择通道"("Enable"=w288) -> ("通道八"=w280:bool, "通道七"=w281:bool, "通道六"=w282:bool, "通道五"=w283:bool, "通道四"=w284:bool, "通道三"=w285:bool, "通道二"=w286:bool, "通道一"=w287:bool)  [unwired: 9 in, 2 out]
                    n168 = Build Array(w287, w286, w285, w284, w283, w282, w281, w280) -> (w279:bool[])
                    n169 = Search 1D Array(1D array=w279, element=TRUE) -> (index of element=w277:i32)  [unwired: 1 in]
                    n170 = local write "通道波形选择 2"(w277) -> ()
                  }
                }
                n171 = case shown="真" w275 {
                  selector: w275 -> [_ w289]
                  frame False {
                  }
                  frame True {
                    n172 = call "请输入滤波模式"("Enable"=w289) -> ("自己选择滤波"=w293:bool, "小波包分解"=w294:bool, "自适应滤波"=w295:bool, "STFT"=w296:bool, "FFT"=w297:bool, "不进行滤波"=w298:bool)  [unwired: 11 in, 2 out]
                    n173 = Build Array(w298, w297, w296, w295, w294, w293) -> (w292:bool[])
                    n174 = Search 1D Array(1D array=w292, element=TRUE) -> (index of element=w290:i32)  [unwired: 1 in]
                    n175 = local write "滤波模式 2"(w290) -> ()
                  }
                }
              }
            }
          }
          frame #1 {
            # "数据滤波"
            n176 = case shown="\"FFT\"" "滤波模式 2" {
              tunnel: w302 -> [w361 w368 _ _ _ w373]
              tunnel: [w361 w367 _ _ _ w372] -> w301
              frame "不进行滤波", Default {
              }
              frame "FFT" {
                n177 = local read "rate"() -> (w363:dbl)
                n178 = call "FFT滤波.vi"("low cutoff freq: fl"="低频截止频率", "high cutoff freq: fh"="高频截止频率", "时域波形图"=w368, "order"="阶数", "filter type"="filter type", "采样频率"=w363) -> ("时域波形图 2"=w367:waveform(dbl)[])
              }
              frame "STFT" {
              }
              frame "自适应滤波" {
              }
              frame "小波包分解" {
              }
              frame "自己设计的滤波方法" {
                n179 = local read "number of samples per channel"() -> (w374:i32)
                n180 = local read "主轴转速"() -> (w376:dbl)
                n181 = Divide(x=w376, y=60.0) -> (x/y=w371:dbl)
                n182 = Multiply(x=w371, y="垂直指针滑动杆") -> (x*y=w369:dbl)
                n183 = call "FFT滤波无mat程序版.vi"("工频频率"=w369, "样本大小"=w374, "时域波形图"=w373) -> ("时域波形图 2"=w372:waveform(dbl)[])
              }
            }
            n184 = case shown="\"幅值\"" "电压&幅值 2" {
              tunnel: w302 -> [w336 w339]
              tunnel: w301 -> [w335 w338]
              tunnel: [w334 w339] -> w300
              tunnel: [w333 w338] -> w299
              frame "电压", Default {
                w337 = "电压（V）"
                n185 = local read "传感器灵敏度"() -> (w332:dbl)
                n186 = local read "传感器灵敏度 2"() -> (w323:dbl)
                n187 = local read "传感器灵敏度 3"() -> (w322:dbl)
                n188 = local read "传感器灵敏度 4"() -> (w321:dbl)
                n189 = local read "传感器灵敏度 5"() -> (w331:dbl)
                n190 = local read "传感器灵敏度 7"() -> (w330:dbl)
                n191 = local read "传感器灵敏度 6"() -> (w329:dbl)
                n192 = local read "传感器灵敏度 8"() -> (w328:dbl)
                n193 = Reciprocal(x=w332) -> (1/x=w320:dbl)
                n194 = Reciprocal(x=w323) -> (1/x=w319:dbl)
                n195 = Reciprocal(x=w322) -> (1/x=w318:dbl)
                n196 = Reciprocal(x=w321) -> (1/x=w317:dbl)
                n197 = Reciprocal(x=w331) -> (1/x=w327:dbl)
                n198 = Reciprocal(x=w330) -> (1/x=w326:dbl)
                n199 = Reciprocal(x=w329) -> (1/x=w325:dbl)
                n200 = Reciprocal(x=w328) -> (1/x=w324:dbl)
                n201 = call "波形倍数.vi"("时域波形图"=w336, "数值"=w320, "数值 5"=w327, "数值 2"=w319, "数值 6"=w326, "数值 3"=w318, "数值 7"=w325, "数值 4"=w317, "数值 8"=w324) -> ("时域波形图 2"=w334:waveform(dbl)[])  [unwired: 10 in]
                n202 = call "波形倍数.vi"("时域波形图"=w335, "数值"=w320, "数值 5"=w327, "数值 2"=w319, "数值 6"=w326, "数值 3"=w318, "数值 7"=w325, "数值 4"=w317, "数值 8"=w324) -> ("时域波形图 2"=w333:waveform(dbl)[])  [unwired: 10 in]
                n203 = property on="滤波前频域信号" class="WFGraph (严格)"("YScale.NameLbl.Text"=w337) -> ()  [unwired: 2 in, 2 out]
                n204 = property on="滤波后时域信号" class="WFGraph (严格)"("YScale.NameLbl.Text"=w337) -> ()  [unwired: 2 in, 2 out]
                n205 = property on="滤波后频域信号" class="WFGraph (严格)"("YScale.NameLbl.Text"=w337) -> ()  [unwired: 2 in, 2 out]
                n206 = property on="滤波前时域信号" class="WFGraph (严格)"("YScale.NameLbl.Text"=w337) -> ()  [unwired: 2 in, 2 out]
              }
              frame "幅值" {
                w340 = "幅值（μm）"
                n207 = property on="滤波前频域信号" class="WFGraph (严格)"("YScale.NameLbl.Text"=w340) -> ()  [unwired: 2 in, 2 out]
                n208 = property on="滤波后时域信号" class="WFGraph (严格)"("YScale.NameLbl.Text"=w340) -> ()  [unwired: 2 in, 2 out]
                n209 = property on="滤波后频域信号" class="WFGraph (严格)"("YScale.NameLbl.Text"=w340) -> ()  [unwired: 2 in, 2 out]
                n210 = property on="滤波前时域信号" class="WFGraph (严格)"("YScale.NameLbl.Text"=w340) -> ()  [unwired: 2 in, 2 out]
              }
            }
            n211 = local read "rate"() -> (w312:dbl)
            n212 = local read "主轴转速"() -> (w311:dbl)
            n213 = Index Array(array=w299, index="通道波形选择 2") -> (element=w314:waveform(dbl))
            "滤波后时域信号" <- w314
            n214 = Index Array(array=w300, index="通道波形选择 2") -> (element=w310:waveform(dbl))
            "滤波前时域信号" <- w310
            n215 = call "转换至动态数据9"("Waveform"=w310) -> ("Dynamic Data Type"=w309:dynamicdata)  [unwired: 3 in]
            n216 = call "从动态数据转换2"("Dynamic Data Type"=w309) -> ("Array"=w308:dbl[])  [unwired: 3 in]
            n217 = script code="Fs;%采样频率\nSpeed;%转速\nfrequence=Speed/60;\ndata=data-mean(data);\nlength_data=length(data);\nfor i=1:1:(length_data)\n    x(i)=sin(2*pi*Speed/60*i/length_data);\n    y(i)=cos(2*pi*Speed/60*i/length_data);\nend\nRdx=0;Rdy=0;\nfor j=1:1:(length_data)\n     m=0;n=0;\n    m=data(j)*x(j);n=data(j)*y(j);\n    Rdx=Rdx+m;Rdy=Rdy+n;\nend\nA=2*(Rdx^2+Rdy^2)^(0.5)/(length_data);\nphase=atan(Rdy/Rdx);\nif Rdx<0\n    phase_ture=phase+pi;\nelse if Rdx>0&&Rdy<0\n        phase_ture=phase+2*pi;\n else \n       phase_ture=phase;\n    end\nend"("Fs"=w312, "Speed"=w311, "data"=w308) -> ("A"=→"工频幅值":dbl, "frequence"=→"工频频率":dbl, "phase_ture"=→"工频相位":dbl)  [unwired: 1 in, 1 out]
            n218 = xnode "频谱测量 3"("信号"=w314) -> ("FFT - （峰值）"=→"滤波后频域信号":cluster{"f0":dbl, "df":dbl, "magnitude":dbl[]})  [unwired: 1 in, 2 out]
            n219 = xnode "频谱测量 2"("信号"=w310) -> ("FFT - （峰值）"=→"滤波前频域信号":cluster{"f0":dbl, "df":dbl, "magnitude":dbl[]})  [unwired: 1 in, 2 out]
            "通道波形选择" <- "通道波形选择 2"
            "滤波模式" <- "滤波模式 2"
          }
          frame #2 {
            # "轴心轨迹绘制"
            n220 = call "通道字符串转换数值常量2.vi"(1:"?") -> ("数值"=w398:i32)
            n221 = call "通道字符串转换数值常量2.vi"(1:"?") -> ("数值"=w397:i32)
            n222 = call "通道字符串转换数值常量2.vi"(1:"?") -> ("数值"=w396:i32)
            n223 = call "通道字符串转换数值常量2.vi"(1:"3") -> ("数值"=w395:i32)
            n224 = Index Array(array=w382, index #1=w398, index #2=w397, index #3=w396, index #4=w395) -> (element #1=w389:waveform(dbl), element #2=w394:waveform(dbl), element #3=w393:waveform(dbl), element #4=w392:waveform(dbl))
            n225 = Merge Signals(w393, w392) -> (w379:dynamicdata)
            n226 = Merge Signals(w389, w394) -> (w380:dynamicdata)
            n227 = Merge Signals(w380, w379) -> (w378:dynamicdata)
            n228 = case shown="真" "保存轴心轨迹数据" {
              selector: "保存轴心轨迹数据" -> [_ w409]
              tunnel: w378 -> [_ w410]
              frame False {
              }
              frame True {
                n229 = call "从动态数据转换5"("Dynamic Data Type"=w410) -> ("Array"=w411:dbl[][])  [unwired: 3 in]
                n230 = call "请选择所需要保存的轴心"("Enable"=w409) -> ("前后端轴心轨迹"=w406:bool, "后端轴心轨迹"=w407:bool, "前端轴心轨迹"=w408:bool)  [unwired: 14 in, 2 out]
                n231 = Build Array(w408, w407, w406) -> (w405:bool[])
                n232 = Search 1D Array(1D array=w405, element=TRUE) -> (index of element=w403:i32)  [unwired: 1 in]
                n233 = stacked-sequence {
                  tunnel: w411 -> [w412 _]
                  tunnel: w403 -> [w414 _]
                  frame #0 {
                    n234 = call "文件对话框2"() -> ("selected path"=w420:path)  [unwired: 12 in, 3 out]
                    n235 = Strip Path(path=w420) -> (stripped path=w416:path, name=w415:string)
                    n236 = Path To String(path=w416) -> (string=w419:string)
                    n237 = Concatenate Strings(w419, "\\" ("字符串"), w415, ".mat" ("字符串")) -> (w413:string)
                    n238 = script code="if a==0||a==1\n   data=data1(1:2,:);\n   save(PATH,'data');\n   else if a==2\n     data=data1(1:4,:);\n     save(PATH,'data');\n   end\nend"("PATH"=w413, "data1"=w412, "a"=w414) -> ()  [unwired: 1 in, 1 out]
                  }
                  frame #1 {
                    n239 = call "显示对话框信息3"("Enable"=TRUE) -> ("确定"=w422:bool)  [unwired: 9 in, 1 out]
                    n240 = Not(x=w422) -> (.not. x?=w421:bool)
                    n241 = local write "保存轴心轨迹数据"(w421) -> ()
                  }
                }
              }
            }
            n242 = call "从动态数据转换3"("Dynamic Data Type"=w380) -> ("Array"=w391:dbl[][])  [unwired: 3 in]
            n243 = call "从动态数据转换4"("Dynamic Data Type"=w379) -> ("Array"=w386:dbl[][])  [unwired: 3 in]
            n244 = Index Array(array=w386) -> (element #1=w384:dbl[], element #2=w385:dbl[])  [unwired: 4 in]
            n245 = Index Array(array=w391) -> (element #1=w388:dbl[], element #2=w390:dbl[])  [unwired: 4 in]
            n246 = Bundle("Array"=w384, "Array"=w385) -> (→"后端实时轴心轨迹":cluster{"Array":dbl[], "Array":dbl[]})  [unwired: 1 in]
            n247 = Bundle("Array"=w388, "Array"=w390) -> (→"前端实时轴心轨迹":cluster{"Array":dbl[], "Array":dbl[]})  [unwired: 1 in]
          }
          frame #3 {
            # "模态分析"
            n248 = case shown="真" "开始 3" {
              frame False {
              }
              frame True {
                n249 = local write "激振计数"(0) -> ()
                n250 = while {
                  shift-right: [w441] -> _
                  shift-left: waveform(dbl)[] [] ("data") -> [w460]
                  tunnel: [w448] -> w432
                  i -> [w444]
                  stop <- w446 stop-if-true
                  w470 = T14 3 items=["无对话框", "确定信息", "继续或停止信息", "确定信息＋警告", "继续/停止+警告"] ("type of dialog (OK msg:1)")
                  # "采集次数"
                  n251 = Greater?(x=w444, y=0) -> (0:w442:bool)
                  n252 = call-poly <vilib>:"DAQmx Create Virtual Channel.vi"("maximum value"="最大采集电压值  2", "minimum value"="最小采集电压值 2", "input terminal configuration"="input terminal configuration 2", "physical channels"="激振信号物理通道", "units"="units 3") -> ("task out"=w476:refnum<k21>, "error out"=w475:errorcluster)  [unwired: 9 in]
                  n253 = call-poly <vilib>:"DAQmx Create Virtual Channel.vi"("task in"=w476, "maximum value"="最大采集电压值  2", "minimum value"="最小采集电压值 2", "input terminal configuration"="input terminal configuration 2", "physical channels"="响应信号物理通道", "units"="units 3", "error in"=w475) -> ("task out"=w467:refnum<k21>, "error out"=w466:errorcluster)  [unwired: 7 in]
                  n254 = Number To Decimal String(number="采集次数") -> (decimal integer string=w438:string)  [unwired: 1 in]
                  n255 = call-poly <vilib>:"DAQmx Timing.vi"("task/channels in"=w467, "sample mode"="sample mode 2", "rate"="rate 2", "error in"=w466) -> ("task out"=w472:refnum<k21>, "error out"=w471:errorcluster)  [unwired: 10 in]
                  n256 = Concatenate Strings("%d /", w438) -> (w437:string)
                  n257 = call <vilib>:"DAQmx Start Task.vi"("task/channels in"=w472, "error in"=w471) -> ("task out"=w463:refnum<k21>, "error out"=w462:errorcluster)  [unwired: 12 in]
                  n258 = property on="激振计数" class="DigNum (严格)"("FormatString"=w437) -> ()  [unwired: 2 in, 2 out]
                  n259 = call-poly <vilib>:"DAQmx Read.vi"("task/channels in"=w463, "number of samples per channel"="number of samples per channel 2", "error in"=w462) -> ("task out"=w458:refnum<k21>, "data"=w441:waveform(dbl)[], "error out"=w459:errorcluster)  [unwired: 10 in]
                  n260 = stacked-sequence {
                    seq-local: [w487 _] -> [_ w535]
                    seq-local: [w486 _] -> [_ w534]
                    seq-local: [w485 _] -> [_ w532]
                    seq-local: [w483 _] -> [_ w533]
                    tunnel: w441 -> [w494 _]
                    tunnel: w460 -> [w495 _]
                    tunnel: w459 -> [w484 _]
                    tunnel: w458 -> [w483 _]
                    tunnel: [_ w531] -> w453
                    tunnel: [_ w524] -> w454
                    tunnel: [_ w528] -> w452
                    tunnel: [_ w527] -> w451
                    tunnel: [_ w526] -> w450
                    tunnel: [_ w525] -> w449
                    tunnel: w442 -> [w481 _]
                    frame #0 {
                      # "现在的问题就就是如何在未达到阈值的时候做处理\n还是有问题 会进入死循环"
                      n261 = Index Array(array=w494, index="激振通道") -> (element=w492:waveform(dbl))
                      n262 = Unbundle By Name(w492) -> ("Y"=w491:dbl[])
                      n263 = Multiply(x=w491, y="激振传感器灵敏度") -> (x*y=w488:dbl[])
                      n264 = Array Max & Min(array=w488) -> (max value=w479:dbl)  [unwired: 3 out]
                      n265 = Absolute Value(x=w479) -> (abs(x)=w478:dbl)
                      n266 = Greater?(x=w478, y="阈值设置") -> (0:w482:bool)
                      n267 = And(x=w482, y=w481) -> (x .and. y?=w480:bool)
                      n268 = case shown="真" w480 {
                        tunnel: w494 -> [_ w509]
                        tunnel: "激振通道" -> [_ w513]
                        tunnel: w484 -> [w499 w510]
                        tunnel: "预触发长度" -> [_ w502]
                        tunnel: w495 -> [w497 w505]
                        tunnel: [w499 w507] -> w485
                        tunnel: [w497 w506] -> w486
                        tunnel: [FALSE TRUE] -> w487
                        frame False {
                        }
                        frame True {
                          w500 = u16 0 items=["采样", "相对时间"] ("start/duration format")
                          n269 = Index Array(array=w509, index=w513) -> (element=w512:waveform(dbl))
                          n270 = call-poly <vilib>:"Number of Waveform Samples.vi"("error in (no error)"=w510, "waveform in"=w512) -> ("error out"=w508:errorcluster, "number of samples"=w511:i32)  [unwired: 7 in, 1 out]
                          n271 = Decrement(x=w511) -> (x-1=w503:i32)
                          n272 = Subtract(x=w503, y=w502) -> (x-y=w501:i32)
                          n273 = for {
                            shift-right: [w518] -> w507
                            shift-left: w508 -> [w523]
                            tunnel: w503 -> [w515]
                            tunnel: w509 -> [w521] mode=indexing
                            tunnel: [w517] -> w506 mode=indexing
                            tunnel: w500 -> [w516]
                            tunnel: w505 -> [w522] mode=indexing
                            tunnel: w501 -> [w514]
                            n274 = call-poly <vilib>:"Append Waveforms.vi"("error in (no error)"=w523, "waveform B"=w521, "waveform A"=w522) -> ("error out"=w519:errorcluster, "waveform out"=w520:waveform(dbl))  [unwired: 7 in]
                            n275 = call-poly <vilib>:"Get Waveform Subset.vi"("start/duration format"=w516, "error in (no error)"=w519, "duration"=w515, "start samples/time"=w514, "waveform in"=w520) -> ("error out"=w518:errorcluster, "waveform out"=w517:waveform(dbl))  [unwired: 1 in, 2 out]
                          }
                        }
                      }
                    }
                    frame #1 {
                      n276 = local read "激振计数"() -> (w529:i32)
                      n277 = call <vilib>:"DAQmx Stop Task.vi"("task/channels in"=w533, "error in"=w532) -> ("task out"=w531:refnum<k21>, "error out"=w530:errorcluster)  [unwired: 12 in]
                      n278 = case shown="真" w535 {
                        tunnel: w534 -> [_ w561]
                        tunnel: w530 -> [w536 w558]
                        tunnel: w529 -> [w537 w560]
                        tunnel: [w537 w559] -> w524
                        tunnel: [w536 w557] -> w528
                        tunnel: [_ w550] -> w527
                        tunnel: [_ w549] -> w526
                        tunnel: [_ w548] -> w525
                        frame False {
                        }
                        frame True {
                          n279 = Index Array(array=w561) -> (element #1=w547:waveform(dbl), element #2=w546:waveform(dbl))  [unwired: 2 in]
                          "激振信号" <- w547
                          n280 = call "单个均值化.vi"("温度信号 4"=w546, "传感器灵敏度"="响应传感器灵敏度") -> ("温度信号 3"=w544:waveform(dbl))
                          n281 = Increment(x=w560) -> (x+1=w559:i32)
                          n282 = Bundle By Name(cluster=T13 {"Topology"=enum."Butterworth", "Type"=enum."Lowpass", "Order"=1, "Lower Fc"=100.0, "Upper Fc"=200.0, "PB Ripple"=1.0, "SB Attenuation"=60.0} ("IIR filter specifications"), "Order"="Order", "Lower Fc"="Lower Fc", "Type"=T12."Lowpass") -> (w541:T13)
                          n283 = call-poly <vilib>:"Digital IIR Filter.vi"("IIR filter specifications"=w541, "signal in"=w544) -> ("signal out"=w543:waveform(dbl))  [unwired: 7 in, 2 out]
                          "响应信号" <- w543
                          n284 = call "平均计算FRF.vi"("time signal X"=w547, "restart averaging (F)"=FALSE, "time signal Y"=w543, "window"="window", "view"="view", "error in (no error)"=w558, "averaging parameters"="averaging parameters", "FRF Mode"="FRF Mode", "删除上一波形"="删除上一次波形") -> ("magnitude"=w550:cluster{"f0":dbl, "df":dbl, "magnitude":dbl[]}, "phase"=w549:cluster{"f0":dbl, "df":dbl, "phase":dbl[]}, "coherence"=w548:cluster{"f0":dbl, "df":dbl, "coherence":dbl[]}, "error out"=w557:errorcluster)  [unwired: 1 in, 2 out]
                        }
                      }
                      n285 = local write "激振计数"(w524) -> ()
                    }
                  }
                  n286 = Greater Or Equal?(x=w454, y="采集次数") -> (x >= y?=w457:bool)
                  n287 = call <vilib>:"DAQmx Clear Task.vi"("task in"=w453, "error in"=w452) -> ("error out"=w469:errorcluster)  [unwired: 13 in]
                  n288 = Select(t=TRUE, s=w457, f=FALSE) -> (s? t:f=w447:bool)
                  n289 = Bundle("magnitude"=w451, "phase"=w450, "coherence"=w449) -> (w448:T15)  [unwired: 1 in]
                  n290 = Or(x=w447, y="停止按钮") -> (x .or. y?=w446:bool)
                  n291 = call <vilib>:"Simple Error Handler.vi"("type of dialog (OK msg:1)"=w470, "error in (no error)"=w469) -> ()  [unwired: 3 in, 5 out]
                }
                n292 = Unbundle(w432) -> ("magnitude"=w430:cluster{"f0":dbl, "df":dbl, "magnitude":dbl[]}, "phase"=w425:cluster{"f0":dbl, "df":dbl, "phase":dbl[]}, "coherence"=→"相关函数":cluster{"f0":dbl, "df":dbl, "coherence":dbl[]})
                "FRF Phase" <- w425
                "FRF magnifitude" <- w430
                n293 = call "模态参数提取（修改的）.vi"("模态阶数"="模态阶数", "FRF Phase"=w425, "FRF magnifitude"=w430) -> ("模态阻尼比"=→"模态阻尼比":dbl[], "模态频率"=→"固有频率":dbl[], "dt"=→"时间间隔":dbl)
              }
            }
          }
        }
      }
      frame "试重平衡" {
        n294 = case shown="真" "开始 2" {
          tunnel: w562 -> [_ w584]
          tunnel: w564 -> [_ w567]
          frame False {
          }
          frame True {
            n295 = call "通道字符串转换数值常量2.vi"(1:"?") -> ("数值"=w579:i32)
            n296 = call "通道字符串转换数值常量2.vi"(1:"?") -> ("数值"=w578:i32)
            n297 = call "通道字符串转换数值常量2.vi"(1:"?") -> ("数值"=w577:i32)
            n298 = call "通道字符串转换数值常量2.vi"(1:"?") -> ("数值"=w585:i32)
            n299 = Index Array(array=w584, index #1=w585, index #2=w579, index #3=w578, index #4=w577) -> (element #1=w571:waveform(dbl), element #2=w570:waveform(dbl), element #3=w569:waveform(dbl), element #4=w568:waveform(dbl))
            n300 = Build Array(w571, w570, w569, w568) -> (w566:waveform(dbl)[])
            n301 = stacked-sequence {
              tunnel: w567 -> [w598 _]
              tunnel: w566 -> [w597 _]
              frame #0 {
                # "0-原始信号\n1-试重信号\n2-配重信号"
                # "求得的工频幅值和相位不断变化"
                n302 = call "通道字符串转换数值常量2.vi"(1:"?") -> ("数值"=w591:i32)
                n303 = call "通道字符串转换数值常量2.vi"(1:"?") -> ("数值"=w592:i32)
                n304 = Build Array("原始信号", "试重信号", "配重信号") -> (w606:bool[])
                n305 = Index Array(array=w597, index #1=w591, index #2=w592) -> (element #1=w596:waveform(dbl), element #2=w595:waveform(dbl))
                n306 = Boolean Array To Number(Boolean array=w606) -> (number=w605:u32)
                n307 = Equal?(x=0, y=w605) -> (x = y?=w603:bool)
                n308 = call "获得信号的最大幅值及对应的相位和频率.vi"("信号"=w595) -> ("max幅值"=w590:dbl, "max相位"=w587:dbl)  [unwired: 2 out]
                n309 = call "获得信号的最大幅值及对应的相位和频率.vi"("信号"=w596) -> ("max幅值"=w589:dbl, "max相位"=w588:dbl)  [unwired: 2 out]
                n310 = case shown="真" w603 {
                  selector: w603 -> [_ w702]
                  tunnel: [w698 w703] -> w608
                  tunnel: w605 -> [w698 _]
                  frame False {
                  }
                  frame True {
                    n311 = call "请选择采集信号类型"("Enable"=w702) -> ("配重信号"=w699:bool, "试重信号"=w700:bool, "原始信号"=w701:bool)  [unwired: 14 in, 2 out]
                    n312 = while {
                      tunnel: [w708] -> w703
                      tunnel: w701 -> [w707]
                      tunnel: w700 -> [w706]
                      tunnel: w699 -> [w705]
                      stop <- w709 continue-if-true
                      n313 = local write "试重信号"(w706) -> ()
                      n314 = Build Array(w707, w706, w705) -> (w710:bool[])
                      n315 = local write "配重信号"(w705) -> ()
                      n316 = local write "原始信号"(w707) -> ()
                      n317 = Boolean Array To Number(Boolean array=w710) -> (number=w708:u32)
                      n318 = Equal?(x=w708, y=0) -> (x = y?=w709:bool)
                    }
                  }
                }
                n319 = To Double Precision Float(number=w608) -> (double precision float=w609:dbl)
                n320 = Logarithm Base 2(1:w609) -> (0:w607:dbl)
                n321 = To Long Integer(number=w607) -> (32bit integer=w599:i32)
                n322 = case shown="0, 默认" w599 {
                  tunnel: w589 -> [w616 w647 w677]
                  tunnel: w590 -> [w617 w646 w676]
                  tunnel: w598 -> [w621 w651 w681]
                  tunnel: w588 -> [w615 w644 w673]
                  tunnel: w587 -> [w612 w641 w670]
                  frame 0, Default {
                    n323 = local read "前端原始信号幅值"() -> (w626:dbl)
                    n324 = local read "计数"() -> (w619:i32)
                    n325 = local read "后端原始信号幅值"() -> (w625:dbl)
                    n326 = Add(x=1, y=w619) -> (x+y=w618:i32)
                    "计数" <- w618
                    n327 = local read "后端原始信号相位"() -> (w611:dbl)
                    n328 = Add(x=w626, y=w616) -> (x+y=w624:dbl)
                    "前端原始信号幅值" <- w624
                    n329 = Add(x=w611, y=w612) -> (x+y=w610:dbl)
                    "后端原始信号相位" <- w610
                    n330 = Add(x=w625, y=w617) -> (x+y=w623:dbl)
                    "后端原始信号幅值" <- w623
                    n331 = Less Or Equal?(x=w618, y=w621) -> (x <= y?=w622:bool)
                    n332 = local read "前端原始信号相位"() -> (w613:dbl)
                    n333 = Add(x=w613, y=w615) -> (x+y=w614:dbl)
                    "前端原始信号相位" <- w614
                    n334 = case shown="真" w622 {
                      tunnel: w624 -> [_ w639]
                      tunnel: w623 -> [_ w638]
                      tunnel: w621 -> [w627 w631]
                      tunnel: w614 -> [_ w635]
                      tunnel: w610 -> [_ w632]
                      frame False {
                        n335 = disable-structure shown="禁用" {
                          disable-tunnel: w627 -> [w628 _]
                          frame Disabled {
                            n336 = local write "计数"(w628) -> ()
                          }
                          frame Enabled {
                          }
                        }
                      }
                      frame True {
                        n337 = Divide(x=w639, y=w631) -> (x/y=w633:dbl)
                        n338 = Divide(x=w638, y=w631) -> (x/y=w630:dbl)
                        n339 = Divide(x=w632, y=w631) -> (x/y=w629:dbl)
                        n340 = Divide(x=w635, y=w631) -> (x/y=w634:dbl)
                        n341 = Polar To Complex(1:w634, 2:w633) -> (0:→"前端原始信号重组":cdb)
                        n342 = Polar To Complex(1:w629, 2:w630) -> (0:→"后端原始信号重组":cdb)
                      }
                    }
                  }
                  frame 1 {
                    n343 = local read "计数 2"() -> (w649:i32)
                    n344 = local read "前端试重信号相位"() -> (w645:dbl)
                    n345 = local read "后端试重信号幅值"() -> (w655:dbl)
                    n346 = local read "后端试重信号相位"() -> (w642:dbl)
                    n347 = local read "前端试重信号幅值"() -> (w656:dbl)
                    n348 = Add(x=1, y=w649) -> (x+y=w648:i32)
                    "计数 2" <- w648
                    n349 = Add(x=w645, y=w644) -> (x+y=w643:dbl)
                    "前端试重信号相位" <- w643
                    n350 = Add(x=w656, y=w647) -> (x+y=w653:dbl)
                    "前端试重信号幅值" <- w653
                    n351 = Add(x=w642, y=w641) -> (x+y=w640:dbl)
                    "后端试重信号相位" <- w640
                    n352 = Add(x=w655, y=w646) -> (x+y=w652:dbl)
                    "后端试重信号幅值" <- w652
                    n353 = Less Or Equal?(x=w648, y=w651) -> (x <= y?=w654:bool)
                    n354 = case shown="假" w654 {
                      tunnel: w653 -> [_ w668]
                      tunnel: w651 -> [w657 w664]
                      tunnel: w652 -> [_ w667]
                      tunnel: w643 -> [_ w666]
                      tunnel: w640 -> [_ w665]
                      frame False {
                        n355 = local write "计数 2"(w657) -> ()
                      }
                      frame True {
                        n356 = Divide(x=w668, y=w664) -> (x/y=w659:dbl)
                        n357 = Divide(x=w667, y=w664) -> (x/y=w663:dbl)
                        n358 = Divide(x=w665, y=w664) -> (x/y=w662:dbl)
                        n359 = Divide(x=w666, y=w664) -> (x/y=w658:dbl)
                        n360 = Polar To Complex(1:w662, 2:w663) -> (0:→"后端试重信号重组":cdb)
                        n361 = Polar To Complex(1:w658, 2:w659) -> (0:→"前端试重信号重组":cdb)
                      }
                    }
                  }
                  frame 2 {
                    n362 = local read "前端配重信号幅值"() -> (w685:dbl)
                    n363 = local read "前端配重信号相位"() -> (w674:dbl)
                    n364 = local read "后端配重信号相位"() -> (w671:dbl)
                    n365 = local read "后端配重信号幅值"() -> (w684:dbl)
                    n366 = local read "计数3"() -> (w679:i32)
                    n367 = Add(x=1, y=w679) -> (x+y=w678:i32)
                    "计数3" <- w678
                    n368 = Add(x=w674, y=w673) -> (x+y=w672:dbl)
                    "前端配重信号相位" <- w672
                    n369 = Add(x=w685, y=w677) -> (x+y=w675:dbl)
                    "前端配重信号幅值" <- w675
                    n370 = Add(x=w671, y=w670) -> (x+y=w669:dbl)
                    "后端配重信号相位" <- w669
                    n371 = Add(x=w684, y=w676) -> (x+y=w682:dbl)
                    "后端配重信号幅值" <- w682
                    n372 = Less Or Equal?(x=w678, y=w681) -> (x <= y?=w683:bool)
                    n373 = case shown="真" w683 {
                      tunnel: w675 -> [_ w697]
                      tunnel: w681 -> [w686 w693]
                      tunnel: w682 -> [_ w696]
                      tunnel: w672 -> [_ w695]
                      tunnel: w669 -> [_ w694]
                      frame False {
                        n374 = local write "计数3"(w686) -> ()
                      }
                      frame True {
                        n375 = Divide(x=w697, y=w693) -> (x/y=w691:dbl)
                        n376 = Divide(x=w696, y=w693) -> (x/y=w689:dbl)
                        n377 = Divide(x=w694, y=w693) -> (x/y=w688:dbl)
                        n378 = Divide(x=w695, y=w693) -> (x/y=w690:dbl)
                        n379 = Polar To Complex(1:w688, 2:w689) -> (0:→"后端配重信号重组":cdb)
                        n380 = Polar To Complex(1:w690, 2:w691) -> (0:→"前端配重信号重组":cdb)
                      }
                    }
                  }
                }
              }
              frame #1 {
                n381 = Build Array("后端", "前端") -> (w715:bool[])
                n382 = Search 1D Array(1D array=w715, element=TRUE) -> (index of element=w718:i32)  [unwired: 1 in]
                n383 = case shown="1" w718 {
                  tunnel: [w731 w734] -> w712
                  tunnel: [w729 w733] -> w713
                  tunnel: [w730 w732] -> w711
                  frame 0, Default {
                    n384 = local read "后端配重信号重组"() -> (w729:cdb)
                    n385 = local read "后端试重信号重组"() -> (w730:cdb)
                    n386 = local read "后端原始信号重组"() -> (w731:cdb)
                  }
                  frame 1 {
                    n387 = local read "前端试重信号重组"() -> (w732:cdb)
                    n388 = local read "前端原始信号重组"() -> (w734:cdb)
                    n389 = local read "前端配重信号重组"() -> (w733:cdb)
                  }
                }
                n390 = case shown="真" "确定计算" {
                  tunnel: w711 -> [_ w741]
                  tunnel: w712 -> [_ w742]
                  frame False {
                  }
                  frame True {
                    n391 = call "单面配重.vi"("f1_weight"="试重重量", "f1_locate"="试重位置", "vibra_f0"=w742, "vibra_f1"=w741, "配重盘孔的数量"="配重盘孔数") -> ("CW_decomp_f_first_weight"=→"第一配重重量":dbl, "CW_decomp_f_first_locate"=→"第一配重位置":dbl, "CW_decomp_f_second_weight"=→"第二配重重量":dbl, "CW_decomp_f_second_locate"=→"第二配重位置":dbl, "err1"=→"配重误差":dbl)  [unwired: 6 in]
                  }
                }
                n392 = Complex To Polar(r * e^(i*theta)=w712) -> (r=→"原始振动幅值":dbl, theta=w725:dbl)
                n393 = Complex To Polar(r * e^(i*theta)=w713) -> (r=→"配重振动幅值":dbl, theta=w723:dbl)
                n394 = Complex To Polar(r * e^(i*theta)=w711) -> (r=→"试重振动幅值":dbl, theta=w720:dbl)
                n395 = expression code="x*180/pi"(w723) -> (→"配重信号相位":dbl)
                n396 = expression code="x*180/pi"(w720) -> (→"试重信号相位":dbl)
                n397 = expression code="x*180/pi"(w725) -> (→"原始信号相位":dbl)
              }
            }
            n398 = call "选择性通道波形显示.vi"("布尔"="?", "布尔 2"="?", "振动信号"=w566, "布尔 3"="?", "布尔 4"="?") -> ("选择性显示通道信号"=w572:waveform(dbl)[])  [unwired: 4 in]
            "时域信号" <- w572
            n399 = xnode "频谱测量"("信号"=w572) -> ("FFT - （峰值）"=→"频域信号":cluster{"f0":dbl, "df":dbl, "magnitude":dbl[]}[])  [unwired: 1 in, 2 out]
            n400 = disable-structure shown="禁用" {
              frame Disabled {
                n401 = local read "前端试重信号重组"() -> ()  [unwired: 1 out]
                n402 = local read "前端原始信号重组"() -> ()  [unwired: 1 out]
              }
              frame Enabled {
              }
            }
          }
        }
      }
    }
  }
  n403 = disable-structure shown="禁用" {
    frame Disabled {
      n404 = case shown="\"电压\", 默认" {
        selector: _ -> [_ _]
        frame "电压", Default {
          w755 = 0.005
          n405 = property on="频域波形图" class="WFGraph (严格)"("YScale.Multiplier"=w755) -> ()  [unwired: 2 in, 2 out]
          n406 = property on="时域波形图" class="WFGraph (严格)"("YScale.Multiplier"=w755) -> ()  [unwired: 2 in, 2 out]
        }
        frame "幅值" {
          w756 = 1.0
          n407 = property on="频域波形图" class="WFGraph (严格)"("YScale.Multiplier"=w756) -> ()  [unwired: 2 in, 2 out]
          n408 = property on="时域波形图" class="WFGraph (严格)"("YScale.Multiplier"=w756) -> ()  [unwired: 2 in, 2 out]
        }
      }
    }
    frame Enabled {
    }
  }
  "布尔" <- FALSE
